vi "TCC.vi"() -> (2 "State out":string="Data: Load Thermal Calibration")   [LabVIEW 2024]
uses:
  DataCluster_TCAL.ctl
  <vilib>/vision/Image Controls.llb/IMAQ Image.ctl
  TCE_Config.ctl
  DataCluster.ctl
  <vilib>/userDefined/High Color/IMAQdx.ctl
  <vilib>/Utility/xml.llb/Write to XML File(string).vi
panel:
  out "OverlayTemp":bool=TRUE
  out "Pict Ring":i32(ring)
  in  "Save":bool
  out "Step":string="Step: 4\n\nCalculate temperature!"
  in  "Fixpoint Radius":i32=20 min=1 max=20
  in  "Cluster":T1={"Core"={"Current VI Reference"=refnum, "Close Panel on Exit?"=FALSE}, "Image Out"=refnum, "State"=0, "Points"={"Top Left"={"X"=0.0, "Y"=0.0}, "Top Right"={"X"=0.0, "Y"=0.0}, "Bottom Left"={"X"=0.0, "Y"=0.0}, "Bottom Right"={"X"=0.0, "Y"=0.0}, "x space 2"=0.0, "y space 2"=0.0, "x_space"=0.0, "y_space"=0.0, "Pixels"=[], "Fixpoint"={"X"=0.0, "Y"=0.0}}, "img_array"=[], "Temps"=[], "Temps_Array"=[], "Scan Area"=0.0, "Fixpoint Area"=0.0, "Config"={"Freezing"={"Cutoff"=2.0, "EndIndex"=2}}, "PCR Size"=0, "ImageCount"=0, "ShowGradient"=FALSE} {"Points"."Bottom Right"."Y" format="%.2f"; "Points"."Bottom Right"."X" format="%.2f"; "Points"."Top Left"."Y" format="%.2f"; "Points"."Top Left"."X" format="%.2f"; "Points"."Top Right"."Y" format="%.2f"; "Points"."Top Right"."X" format="%.2f"; "Points"."Bottom Left"."Y" format="%.2f"; "Points"."Bottom Left"."X" format="%.2f"; "Points"."Fixpoint"."Y" format="%.2f"; "Points"."Fixpoint"."X" format="%.2f"}
  in  "Display Mapping":u32(ring)=10 items=["Default"=10, "Most Significant Bits"=11, "Full Dynamic"=12, "Downshift"=13, "Given Range"=14, "90% Dynamic"=15, "Given Percent Range"=16]
  in  "Image":u32(slide) scale=0.0..242.0
  in  "Help":bool
  out "Tutorial":string="Step: 4\n\nCalculate temperature!"
  in  "Show All Points":bool
  in  "Well Radius":u32=50 min=1 max=100
  in  "PCR Size":u16(ring) items=["384 (24x16)", "96 (12x8)"]
  out "Points":T3[](array[typedef])=[{"X"=103.0, "Y"=94.0}, {"X"=158.04349, "Y"=93.521736}, {"X"=213.08696, "Y"=93.04348}, {"X"=268.13043, "Y"=92.565216}, {"X"=323.17392, "Y"=92.08696}, {"X"=378.2174, "Y"=91.608696}, {"X"=433.26086, "Y"=91.13043}, {"X"=488.30435, "Y"=90.652176}, {"X"=543.34784, "Y"=90.17391}, {"X"=598.39136, "Y"=89.69565}, {"X"=653.4348, "Y"=89.21739}, {"X"=708.4783, "Y"=88.73913}, {"X"=763.5217, "Y"=88.26087}, {"X"=818.56525, "Y"=87.78261}, {"X"=873.6087, "Y"=87.30435}, {"X"=928.6522, "Y"=86.82609}, {"X"=983.6957, "Y"=86.347824}, {"X"=1038.7391, "Y"=85.86957}, {"X"=1093.7827, "Y"=85.391304}, {"X"=1148.8262, "Y"=84.91304}, {"X"=1203.8696, "Y"=84.434784}, {"X"=1258.9131, "Y"=83.95652}, {"X"=1313.9565, "Y"=83.478264}, {"X"=1369.0, "Y"=83.0}, {"X"=103.46667, "Y"=149.06667}, {"X"=158.51015, "Y"=148.58841}, {"X"=213.55362, "Y"=148.11014}, {"X"=268.5971, "Y"=147.63188}, {"X"=323.6406, "Y"=147.15363}, {"X"=378.68408, "Y"=146.67535}, {"X"=433.72754, "Y"=146.1971}, {"X"=488.77103, "Y"=145.71884}, {"X"=543.8145, "Y"=145.24057}, {"X"=598.858, "Y"=144.76231}, {"X"=653.9015, "Y"=144.28406}, {"X"=708.94495, "Y"=143.8058}, {"X"=763.9884, "Y"=143.32753}, {"X"=819.0319, "Y"=142.84927}, {"X"=874.0754, "Y"=142.37102}, {"X"=929.1189, "Y"=141.89276}, {"X"=984.16235, "Y"=141.41449}, {"X"=1039.2058, "Y"=140.93623}, {"X"=1094.2493, "Y"=140.45798}, {"X"=1149.2928, "Y"=139.9797}, {"X"=1204.3363, "Y"=139.50145}, {"X"=1259.3798, "Y"=139.0232}, {"X"=1314.4232, "Y"=138.54492}, {"X"=1369.4667, "Y"=138.06667}, {"X"=103.933334, "Y"=204.13333}, {"X"=158.9768, "Y"=203.65506}, {"X"=214.0203, "Y"=203.17682}, {"X"=269.06375, "Y"=202.69855}, {"X"=324.10724, "Y"=202.22029}, {"X"=379.15073, "Y"=201.74203}, {"X"=434.19418, "Y"=201.26376}, {"X"=489.23767, "Y"=200.7855}, {"X"=544.2812, "Y"=200.30725}, {"X"=599.32465, "Y"=199.82898}, {"X"=654.36816, "Y"=199.35072}, {"X"=709.4116, "Y"=198.87247}, {"X"=764.4551, "Y"=198.3942}, {"X"=819.4986, "Y"=197.91594}, {"X"=874.54205, "Y"=197.43768}, {"X"=929.5856, "Y"=196.95941}, {"X"=984.629, "Y"=196.48116}, {"X"=1039.6725, "Y"=196.0029}, {"X"=1094.716, "Y"=195.52463}, {"X"=1149.7595, "Y"=195.04637}, {"X"=1204.803, "Y"=194.56812}, {"X"=1259.8464, "Y"=194.08984}, {"X"=1314.8899, "Y"=193.6116}, {"X"=1369.9333, "Y"=193.13333}, {"X"=104.4, "Y"=259.2}, {"X"=159.44348, "Y"=258.72174}, {"X"=214.48695, "Y"=258.24347}, {"X"=269.53043, "Y"=257.7652}, {"X"=324.5739, "Y"=257.28696}, {"X"=379.6174, "Y"=256.8087}, {"X"=434.66086, "Y"=256.33044}, {"X"=489.70435, "Y"=255.85217}, {"X"=544.74786, "Y"=255.37392}, {"X"=599.7913, "Y"=254.89565}, {"X"=654.83484, "Y"=254.41739}, {"X"=709.8783, "Y"=253.93913}, {"X"=764.92175, "Y"=253.46086}, {"X"=819.9653, "Y"=252.9826}, {"X"=875.0087, "Y"=252.50435}, {"X"=930.05225, "Y"=252.02608}, {"X"=985.0957, "Y"=251.54782}, {"X"=1040.1392, "Y"=251.06956}, {"X"=1095.1826, "Y"=250.59131}, {"X"=1150.2262, "Y"=250.11304}, {"X"=1205.2697, "Y"=249.63478}, {"X"=1260.3131, "Y"=249.15652}, {"X"=1315.3566, "Y"=248.67825}, {"X"=1370.4, "Y"=248.2}, {"X"=104.86667, "Y"=314.26666}, {"X"=159.91014, "Y"=313.7884}, {"X"=214.95363, "Y"=313.31012}, {"X"=269.9971, "Y"=312.83188}, {"X"=325.0406, "Y"=312.35364}, {"X"=380.08408, "Y"=311.87537}, {"X"=435.12753, "Y"=311.3971}, {"X"=490.17102, "Y"=310.91882}, {"X"=545.2145, "Y"=310.44058}, {"X"=600.258, "Y"=309.9623}, {"X"=655.30145, "Y"=309.48407}, {"X"=710.3449, "Y"=309.0058}, {"X"=765.38837, "Y"=308.52753}, {"X"=820.4319, "Y"=308.04926}, {"X"=875.47534, "Y"=307.571}, {"X"=930.51886, "Y"=307.09274}, {"X"=985.5623, "Y"=306.6145}, {"X"=1040.6058, "Y"=306.13623}, {"X"=1095.6493, "Y"=305.65796}, {"X"=1150.6929, "Y"=305.1797}, {"X"=1205.7363, "Y"=304.70145}, {"X"=1260.7798, "Y"=304.2232}, {"X"=1315.8232, "Y"=303.74493}, {"X"=1370.8667, "Y"=303.26666}, {"X"=105.333336, "Y"=369.3333}, {"X"=160.37682, "Y"=368.85504}, {"X"=215.42029, "Y"=368.3768}, {"X"=270.46378, "Y"=367.89853}, {"X"=325.50726, "Y"=367.42026}, {"X"=380.55075, "Y"=366.94202}, {"X"=435.5942, "Y"=366.46375}, {"X"=490.6377, "Y"=365.98547}, {"X"=545.68115, "Y"=365.50723}, {"X"=600.7247, "Y"=365.02896}, {"X"=655.7681, "Y"=364.5507}, {"X"=710.8116, "Y"=364.07245}, {"X"=765.85504, "Y"=363.59418}, {"X"=820.89856, "Y"=363.11594}, {"X"=875.942, "Y"=362.63766}, {"X"=930.98553, "Y"=362.1594}, {"X"=986.029, "Y"=361.68115}, {"X"=1041.0725, "Y"=361.20288}, {"X"=1096.116, "Y"=360.7246}, {"X"=1151.1595, "Y"=360.24637}, {"X"=1206.203, "Y"=359.7681}, {"X"=1261.2465, "Y"=359.28983}, {"X"=1316.2899, "Y"=358.81158}, {"X"=1371.3334, "Y"=358.3333}, {"X"=105.8, "Y"=424.4}, {"X"=160.84348, "Y"=423.92172}, {"X"=215.88696, "Y"=423.44348}, {"X"=270.93042, "Y"=422.9652}, {"X"=325.9739, "Y"=422.48694}, {"X"=381.0174, "Y"=422.0087}, {"X"=436.06085, "Y"=421.53043}, {"X"=491.10434, "Y"=421.05215}, {"X"=546.1478, "Y"=420.5739}, {"X"=601.19135, "Y"=420.09564}, {"X"=656.2348, "Y"=419.61737}, {"X"=711.27826, "Y"=419.13913}, {"X"=766.3217, "Y"=418.66086}, {"X"=821.36523, "Y"=418.18262}, {"X"=876.4087, "Y"=417.70435}, {"X"=931.4522, "Y"=417.22607}, {"X"=986.49567, "Y"=416.74783}, {"X"=1041.5392, "Y"=416.26956}, {"X"=1096.5826, "Y"=415.7913}, {"X"=1151.6262, "Y"=415.31305}, {"X"=1206.6697, "Y"=414.83478}, {"X"=1261.7131, "Y"=414.3565}, {"X"=1316.7566, "Y"=413.87827}, {"X"=1371.8, "Y"=413.4}, {"X"=106.26667, "Y"=479.46667}, {"X"=161.31015, "Y"=478.9884}, {"X"=216.35362, "Y"=478.51016}, {"X"=271.3971, "Y"=478.0319}, {"X"=326.44058, "Y"=477.55362}, {"X"=381.48407, "Y"=477.07538}, {"X"=436.52753, "Y"=476.5971}, {"X"=491.571, "Y"=476.11884}, {"X"=546.6145, "Y"=475.6406}, {"X"=601.658, "Y"=475.16232}, {"X"=656.7015, "Y"=474.68405}, {"X"=711.74493, "Y"=474.2058}, {"X"=766.7884, "Y"=473.72754}, {"X"=821.8319, "Y"=473.2493}, {"X"=876.87537, "Y"=472.77103}, {"X"=931.9189, "Y"=472.29276}, {"X"=986.96234, "Y"=471.8145}, {"X"=1042.0059, "Y"=471.33624}, {"X"=1097.0493, "Y"=470.85797}, {"X"=1152.0929, "Y"=470.37973}, {"X"=1207.1364, "Y"=469.90146}, {"X"=1262.1798, "Y"=469.4232}, {"X"=1317.2233, "Y"=468.94495}, {"X"=1372.2667, "Y"=468.46667}, {"X"=106.73333, "Y"=534.5333}, {"X"=161.77681, "Y"=534.05505}, {"X"=216.8203, "Y"=533.5768}, {"X"=271.86377, "Y"=533.0985}, {"X"=326.90726, "Y"=532.62024}, {"X"=381.95074, "Y"=532.142}, {"X"=436.9942, "Y"=531.66376}, {"X"=492.0377, "Y"=531.1855}, {"X"=547.0812, "Y"=530.7073}, {"X"=602.12463, "Y"=530.229}, {"X"=657.16815, "Y"=529.75073}, {"X"=712.2116, "Y"=529.27246}, {"X"=767.25507, "Y"=528.7942}, {"X"=822.2986, "Y"=528.3159}, {"X"=877.34204, "Y"=527.83765}, {"X"=932.38556, "Y"=527.3594}, {"X"=987.429, "Y"=526.88116}, {"X"=1042.4724, "Y"=526.4029}, {"X"=1097.516, "Y"=525.9246}, {"X"=1152.5594, "Y"=525.4464}, {"X"=1207.6029, "Y"=524.96814}, {"X"=1262.6464, "Y"=524.48987}, {"X"=1317.6898, "Y"=524.0116}, {"X"=1372.7333, "Y"=523.5333}, {"X"=107.2, "Y"=589.6}, {"X"=162.24348, "Y"=589.1217}, {"X"=217.28696, "Y"=588.64343}, {"X"=272.33044, "Y"=588.16516}, {"X"=327.37393, "Y"=587.6869}, {"X"=382.41742, "Y"=587.2087}, {"X"=437.46088, "Y"=586.7304}, {"X"=492.50436, "Y"=586.25214}, {"X"=547.54785, "Y"=585.7739}, {"X"=602.5913, "Y"=585.29565}, {"X"=657.6348, "Y"=584.8174}, {"X"=712.6783, "Y"=584.3391}, {"X"=767.72174, "Y"=583.86084}, {"X"=822.76526, "Y"=583.38257}, {"X"=877.8087, "Y"=582.9043}, {"X"=932.85223, "Y"=582.426}, {"X"=987.8957, "Y"=581.9478}, {"X"=1042.9391, "Y"=581.46954}, {"X"=1097.9827, "Y"=580.9913}, {"X"=1153.0261, "Y"=580.51306}, {"X"=1208.0696, "Y"=580.0348}, {"X"=1263.113, "Y"=579.5565}, {"X"=1318.1565, "Y"=579.07825}, {"X"=1373.2, "Y"=578.6}, {"X"=107.666664, "Y"=644.6666}, {"X"=162.71014, "Y"=644.18835}, {"X"=217.75363, "Y"=643.7101}, {"X"=272.7971, "Y"=643.2319}, {"X"=327.84058, "Y"=642.7536}, {"X"=382.88406, "Y"=642.2753}, {"X"=437.92752, "Y"=641.79706}, {"X"=492.971, "Y"=641.3188}, {"X"=548.0145, "Y"=640.8405}, {"X"=603.058, "Y"=640.3623}, {"X"=658.1015, "Y"=639.88403}, {"X"=713.14496, "Y"=639.40576}, {"X"=768.1884, "Y"=638.9275}, {"X"=823.23193, "Y"=638.4492}, {"X"=878.2754, "Y"=637.97095}, {"X"=933.3189, "Y"=637.49274}, {"X"=988.36237, "Y"=637.01447}, {"X"=1043.4058, "Y"=636.5362}, {"X"=1098.4493, "Y"=636.0579}, {"X"=1153.4928, "Y"=635.57965}, {"X"=1208.5363, "Y"=635.1014}, {"X"=1263.5797, "Y"=634.62317}, {"X"=1318.6232, "Y"=634.1449}, {"X"=1373.6666, "Y"=633.6666}, {"X"=108.13333, "Y"=699.73334}, {"X"=163.17682, "Y"=699.25507}, {"X"=218.22029, "Y"=698.7768}, {"X"=273.26376, "Y"=698.2986}, {"X"=328.30725, "Y"=697.8203}, {"X"=383.35074, "Y"=697.34204}, {"X"=438.3942, "Y"=696.8638}, {"X"=493.43768, "Y"=696.3855}, {"X"=548.4812, "Y"=695.9072}, {"X"=603.52466, "Y"=695.429}, {"X"=658.5682, "Y"=694.95074}, {"X"=713.61163, "Y"=694.4725}, {"X"=768.6551, "Y"=693.9942}, {"X"=823.6986, "Y"=693.5159}, {"X"=878.74207, "Y"=693.03766}, {"X"=933.7856, "Y"=692.55945}, {"X"=988.82904, "Y"=692.0812}, {"X"=1043.8724, "Y"=691.6029}, {"X"=1098.916, "Y"=691.12463}, {"X"=1153.9595, "Y"=690.64636}, {"X"=1209.0029, "Y"=690.1681}, {"X"=1264.0464, "Y"=689.6899}, {"X"=1319.0898, "Y"=689.2116}, {"X"=1374.1333, "Y"=688.73334}, {"X"=108.6, "Y"=754.8}, {"X"=163.64348, "Y"=754.3217}, {"X"=218.68697, "Y"=753.84344}, {"X"=273.73044, "Y"=753.36523}, {"X"=328.77393, "Y"=752.88696}, {"X"=383.8174, "Y"=752.4087}, {"X"=438.86087, "Y"=751.9304}, {"X"=493.90436, "Y"=751.45215}, {"X"=548.9478, "Y"=750.9739}, {"X"=603.99133, "Y"=750.49567}, {"X"=659.0348, "Y"=750.0174}, {"X"=714.07825, "Y"=749.5391}, {"X"=769.1217, "Y"=749.06085}, {"X"=824.1652, "Y"=748.5826}, {"X"=879.2087, "Y"=748.1043}, {"X"=934.2522, "Y"=747.6261}, {"X"=989.29565, "Y"=747.1478}, {"X"=1044.3391, "Y"=746.66956}, {"X"=1099.3827, "Y"=746.1913}, {"X"=1154.4261, "Y"=745.713}, {"X"=1209.4696, "Y"=745.23474}, {"X"=1264.5131, "Y"=744.75653}, {"X"=1319.5565, "Y"=744.27826}, {"X"=1374.6, "Y"=743.8}, {"X"=109.066666, "Y"=809.86664}, {"X"=164.11015, "Y"=809.38837}, {"X"=219.15363, "Y"=808.9101}, {"X"=274.1971, "Y"=808.4319}, {"X"=329.2406, "Y"=807.9536}, {"X"=384.2841, "Y"=807.47534}, {"X"=439.32755, "Y"=806.9971}, {"X"=494.37103, "Y"=806.5188}, {"X"=549.4145, "Y"=806.0405}, {"X"=604.458, "Y"=805.5623}, {"X"=659.50146, "Y"=805.08405}, {"X"=714.5449, "Y"=804.6058}, {"X"=769.5884, "Y"=804.1275}, {"X"=824.6319, "Y"=803.64923}, {"X"=879.67535, "Y"=803.17096}, {"X"=934.7189, "Y"=802.69275}, {"X"=989.7623, "Y"=802.2145}, {"X"=1044.8058, "Y"=801.7362}, {"X"=1099.8494, "Y"=801.25793}, {"X"=1154.8928, "Y"=800.77966}, {"X"=1209.9363, "Y"=800.3014}, {"X"=1264.9797, "Y"=799.8232}, {"X"=1320.0232, "Y"=799.3449}, {"X"=1375.0667, "Y"=798.86664}, {"X"=109.53333, "Y"=864.93335}, {"X"=164.57681, "Y"=864.4551}, {"X"=219.6203, "Y"=863.9768}, {"X"=274.66376, "Y"=863.4986}, {"X"=329.70724, "Y"=863.0203}, {"X"=384.75073, "Y"=862.54205}, {"X"=439.7942, "Y"=862.0638}, {"X"=494.83768, "Y"=861.5855}, {"X"=549.88116, "Y"=861.10724}, {"X"=604.9247, "Y"=860.629}, {"X"=659.96814, "Y"=860.15076}, {"X"=715.0116, "Y"=859.6725}, {"X"=770.05505, "Y"=859.1942}, {"X"=825.0986, "Y"=858.71594}, {"X"=880.142, "Y"=858.2377}, {"X"=935.18555, "Y"=857.75946}, {"X"=990.229, "Y"=857.2812}, {"X"=1045.2725, "Y"=856.8029}, {"X"=1100.316, "Y"=856.32465}, {"X"=1155.3595, "Y"=855.8464}, {"X"=1210.403, "Y"=855.3681}, {"X"=1265.4464, "Y"=854.8899}, {"X"=1320.4899, "Y"=854.4116}, {"X"=1375.5333, "Y"=853.93335}, {"X"=110.0, "Y"=920.0}, {"X"=165.04349, "Y"=919.5217}, {"X"=220.08696, "Y"=919.04346}, {"X"=275.13043, "Y"=918.56525}, {"X"=330.17392, "Y"=918.087}, {"X"=385.2174, "Y"=917.6087}, {"X"=440.26086, "Y"=917.13043}, {"X"=495.30435, "Y"=916.65216}, {"X"=550.34784, "Y"=916.1739}, {"X"=605.39136, "Y"=915.6957}, {"X"=660.4348, "Y"=915.2174}, {"X"=715.4783, "Y"=914.73914}, {"X"=770.5217, "Y"=914.26086}, {"X"=825.56525, "Y"=913.7826}, {"X"=880.6087, "Y"=913.3043}, {"X"=935.6522, "Y"=912.8261}, {"X"=990.6957, "Y"=912.34784}, {"X"=1045.7391, "Y"=911.86957}, {"X"=1100.7827, "Y"=911.3913}, {"X"=1155.8262, "Y"=910.913}, {"X"=1210.8696, "Y"=910.43475}, {"X"=1265.9131, "Y"=909.95654}, {"X"=1320.9565, "Y"=909.4783}, {"X"=1376.0, "Y"=909.0}] {"Y" format="%.2f"; "X" format="%.2f"}
  out "State":i32=3
  in  "Previous":bool
  in  "Next":bool
  in  "Path":path caption="Image Path"
  out "Image":T2(plugin-control)
  # "hints \nPress F1 or F2 to cycle through the steps\nUse the Mouse Wheel to zoom in and out"
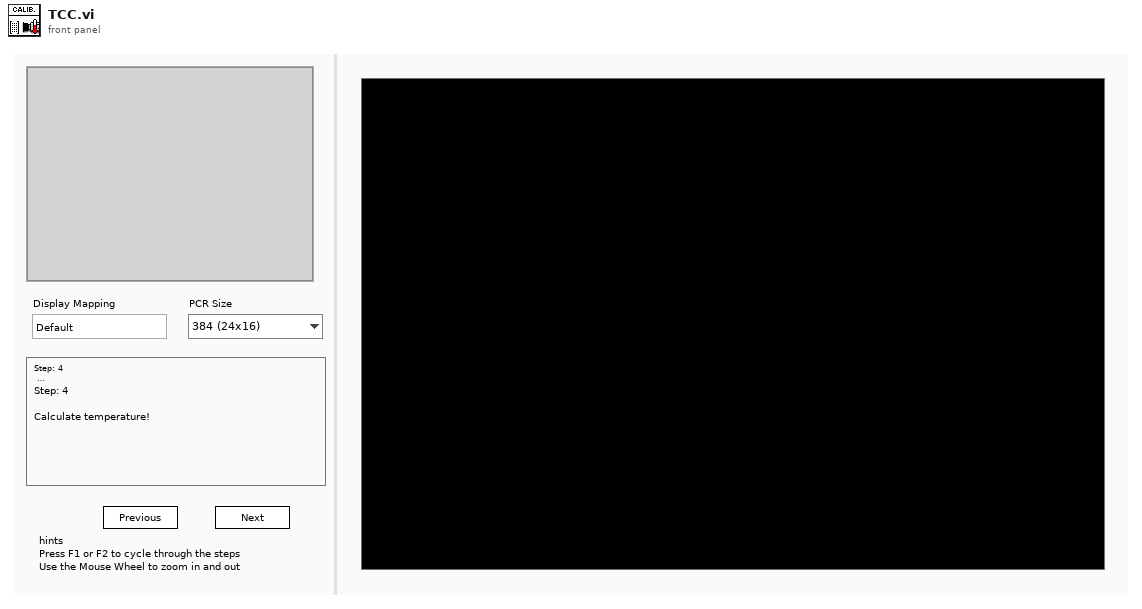
[diagram p1: front panel]
types:
  T1 = typedef "DataCluster_TCAL.ctl" = cluster{"Core":cluster{"Current VI Reference":refnum<vi>, "Close Panel on Exit?":bool}, "Image Out":T2, "State":i32, "Points":cluster{"Top Left":T3, "Top Right":T3, "Bottom Left":T3, "Bottom Right":T3, "x space 2":dbl, "y space 2":sgl, "x_space":sgl, "y_space":sgl, "Pixels":cluster{"X":i32, "Y":i32}[][], "Fixpoint":T3}, "img_array":T2[], "Temps":dbl[], "Temps_Array":dbl[][], "Scan Area":dbl, "Fixpoint Area":dbl, "Config":T4, "PCR Size":u16, "ImageCount":i32, "ShowGradient":bool}
  T2 = typedef "IMAQ Image.ctl" = refnum<image>
  T3 = typedef "IMAQ Point" = cluster{"X":sgl, "Y":sgl}
  T4 = typedef "TCE_Config.ctl" = cluster{"Freezing":cluster{"Cutoff":dbl, "EndIndex":i32}}
  T5 = enum32{"Invalid", "Standard", "Closed", "Hidden", "Minimized", "Maximized"}
  T6 = enum32{"invalid app kind", "Development System", "Run Time System", "Student Edition", "Embedded LabVIEW", "Evaluation", "Custom"}
  T7 = cluster{"Global Rectangle":i32[], "Contours":cluster{"Contour Type":u32, "ROI Type":u32, "Points":i32[]}[]}
  T8 = typedef "DataCluster.ctl" = cluster{"Core":cluster{"Current VI Reference":refnum<vi>, "Close Panel on Exit?":bool, "Exit":bool, "Initialized?":bool}, "Connections":cluster{"cDAQ":cluster{"Task":refnum<k21>, "Connected":bool, "Active":bool, "ID":string}, "Camera":cluster{"Session":T9, "Connected":bool, "Active":bool, "Placeholder":T2}, "PSU":cluster{"Port":refnum<visa-resource-name>, "Connected":bool, "Active":bool}, "Arduino":cluster{"Port":refnum<visa-resource-name>, "Connected":bool, "Active":bool}}, "Data Acquisition":cluster{"Setup":cluster{"Label":string, "Operator":string, "Notes":string, "TempGrad":dbl, "TargetTemp":dbl, "Sample Volume":dbl}, "Camera":cluster{"Image":T2, "Save Image":T2, "Image Frequency":i32, "Rectangle":T10, "Calibration":cluster{"Top Left":T3, "Top Right":T3, "Bottom Left":T3, "Bottom Right":T3, "Fixpoint":T3, "Scan Area":dbl, "Fixpoint Area":dbl, "Well Pixels":cluster{"X":i32, "Y":i32}[][], "Valid":bool}, "FocusPos":u32, "Display Mapping":u32, "Camera Mode":u32}, "Thermistor":cluster{"Sample Size":i32, "Calibration":cluster{"B0.100":dbl[], "R25":dbl[], "c":dbl[][], "State":bool[], "V_S":dbl, "R_S":dbl}, "Timing Mode":i32}, "Partition":cluster{"Data":string[][], "Cell Label":string, "Cell Color":u32, "Height":i32, "Width":i32, "Grid":string[][]}, "Queue":cluster{"Size":i32, "Queue":refnum<queue>}, "Sample Rate":i32, "Active":bool, "Ready":bool, "Graph Mode":u16, "Gradient Buffer":i32}, "Control":cluster{"Sample Rate":i32, "PID gains":cluster{"proportional gain (Kc)":dbl, "integral time (Ti, min)":dbl, "derivative time (Td, min)":dbl}}, "Manual Temp Control":cluster{"TargetTemp":dbl, "Mode":u16, "Active":bool}}
  T9 = typedef "IMAQdx.ctl" = refnum<k21>
  T10 = typedef "IMAQ Rectangle" = cluster{"Left":i32, "Top":i32, "Right":i32, "Bottom":i32, "Rotation":dbl}
  T11 = enum16{"open", "replace", "create", "open or create", "replace or create", "replace or create with confirmation"}
  T12 = typedef "ROI Descriptor" = cluster{"Global Rectangle":i32[], "Contours":cluster{"ID":enum32{"External", "Internal"}, "Type":u32, "Coordinates":i32[]}[]}
  T13 = typedef "Image Type" = u32
  T14 = cluster{"Current VI Reference":refnum<vi>, "Close Panel on Exit?":bool}
  T15 = cluster{"Top Left":T3, "Top Right":T3, "Bottom Left":T3, "Bottom Right":T3, "x space 2":dbl, "y space 2":sgl, "x_space":sgl, "y_space":sgl, "Pixels":cluster{"X":i32, "Y":i32}[][], "Fixpoint":T3}
  T16 = cluster{"Top Left":T3, "Top Right":T3, "Bottom Left":T3, "Bottom Right":T3, "Fixpoint":T3, "Scan Area":dbl, "Fixpoint Area":dbl, "Well Pixels":cluster{"X":i32, "Y":i32}[][], "Valid":bool}
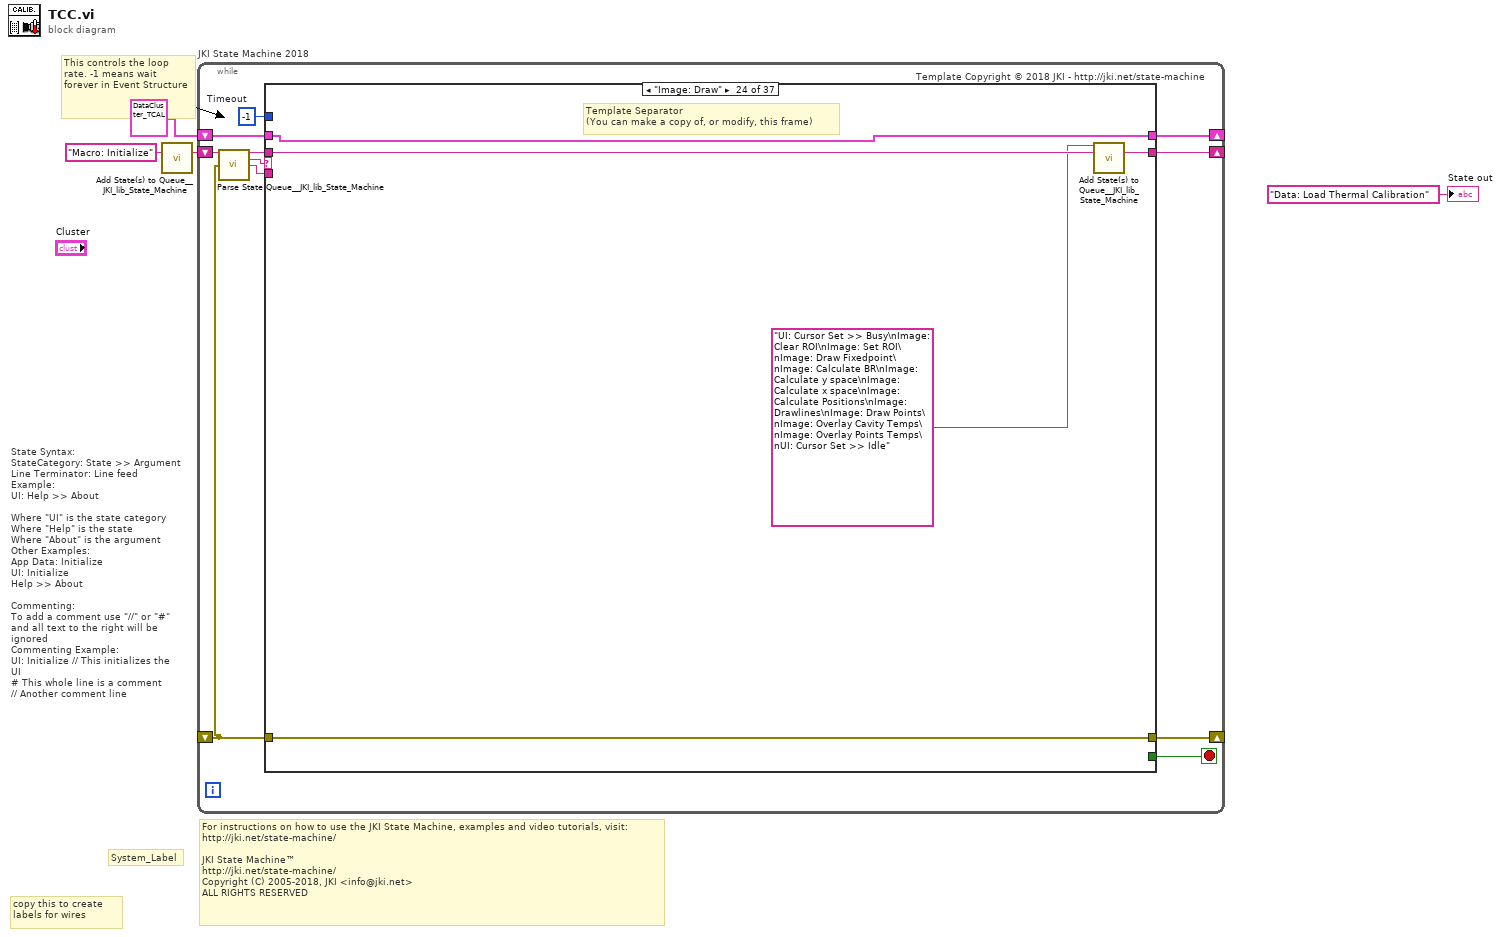
[diagram p0: block diagram]
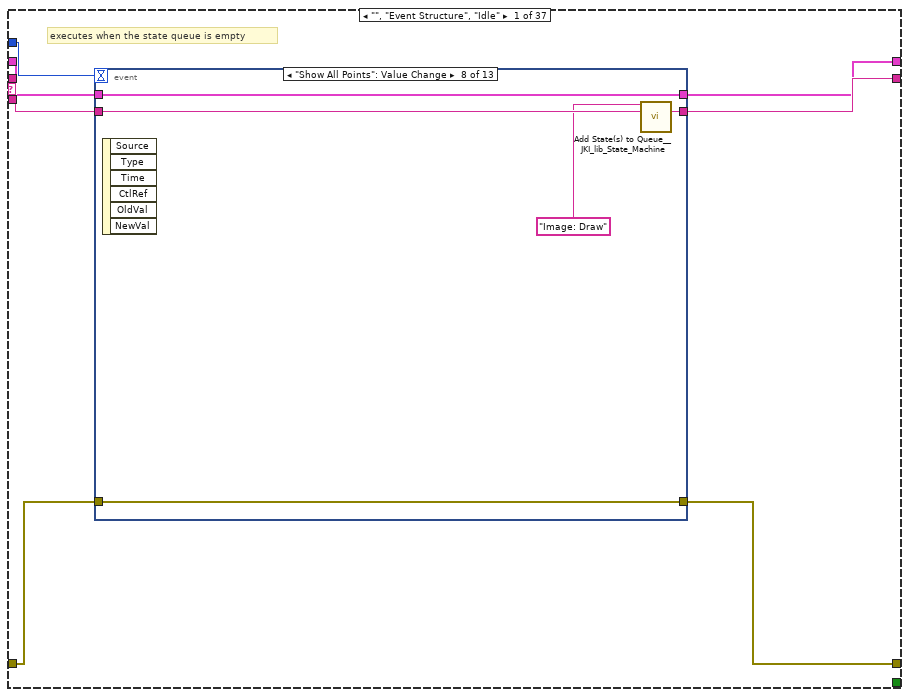
[diagram p2: hidden frame]
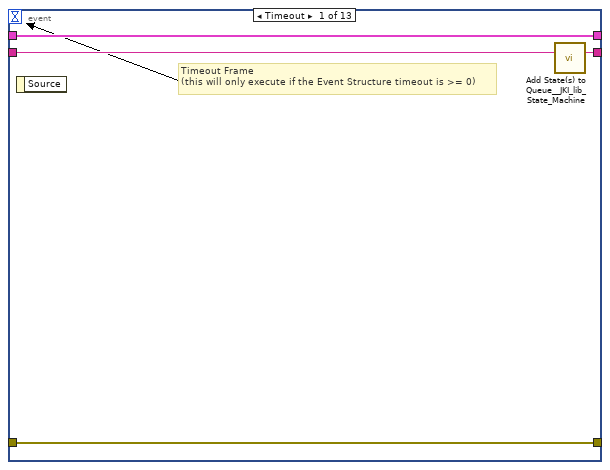
[diagram p3: hidden frame]
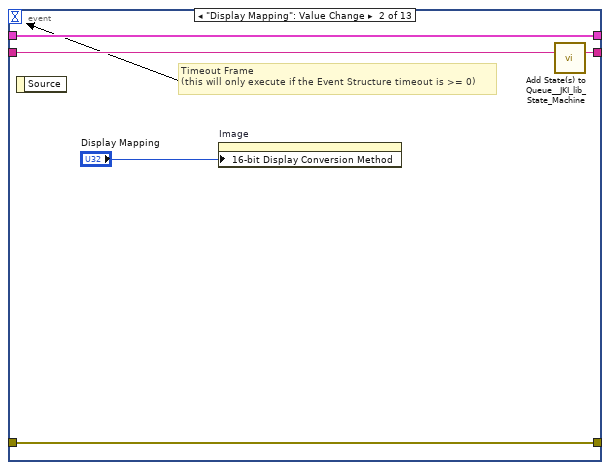
[diagram p4: hidden frame]
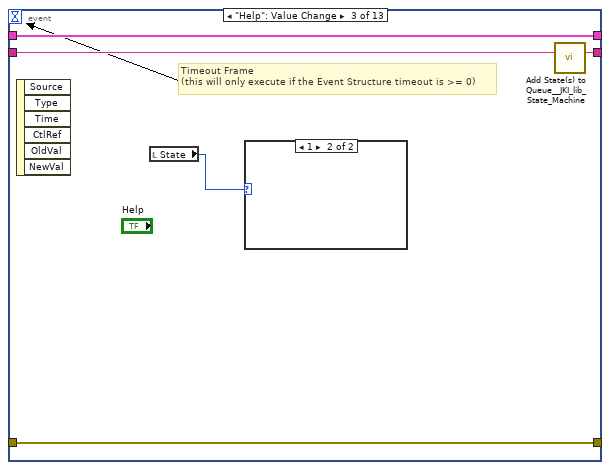
[diagram p5: hidden frame]
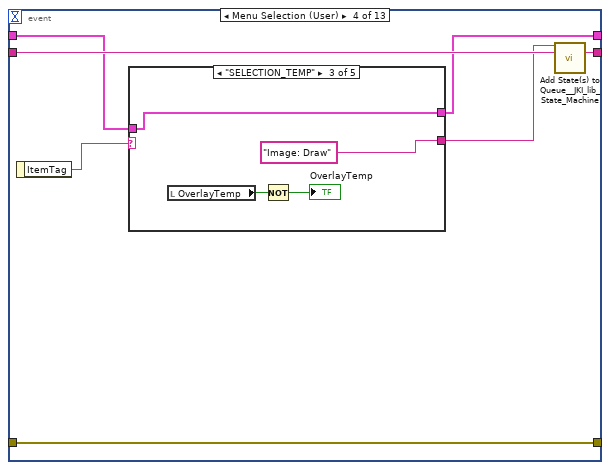
[diagram p7: hidden frame]
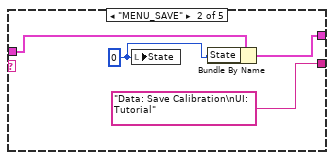
[diagram p9: hidden frame]
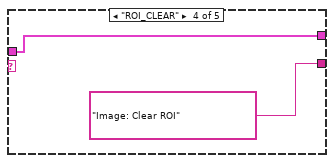
[diagram p10: hidden frame]
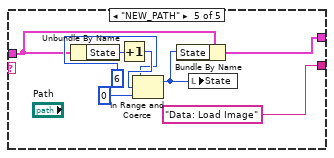
[diagram p11: hidden frame]
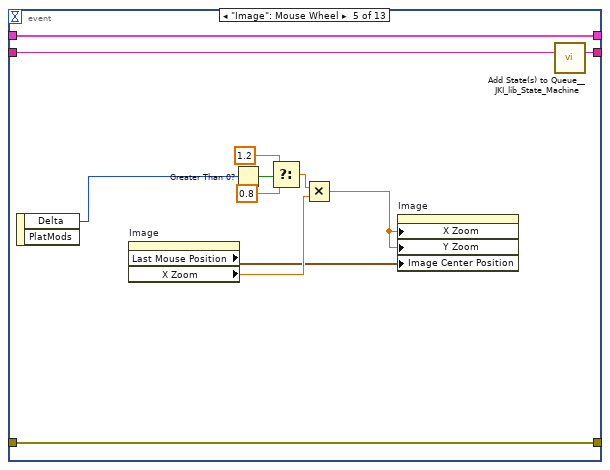
[diagram p12: hidden frame]
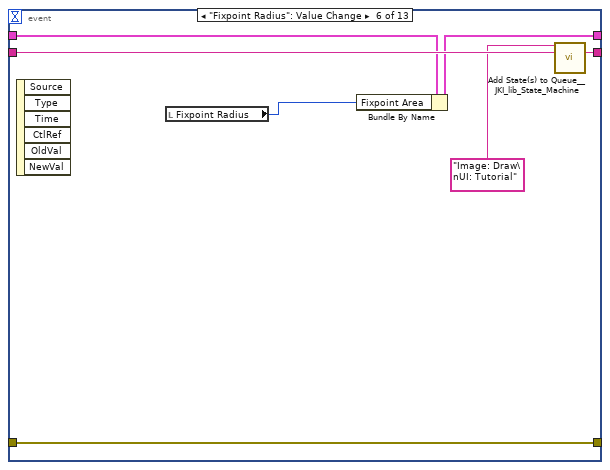
[diagram p13: hidden frame]
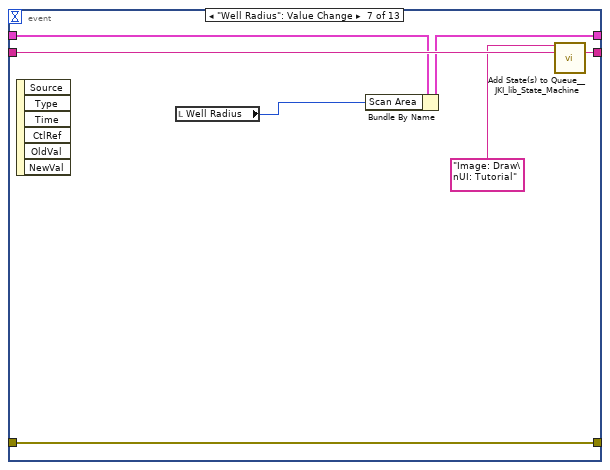
[diagram p14: hidden frame]
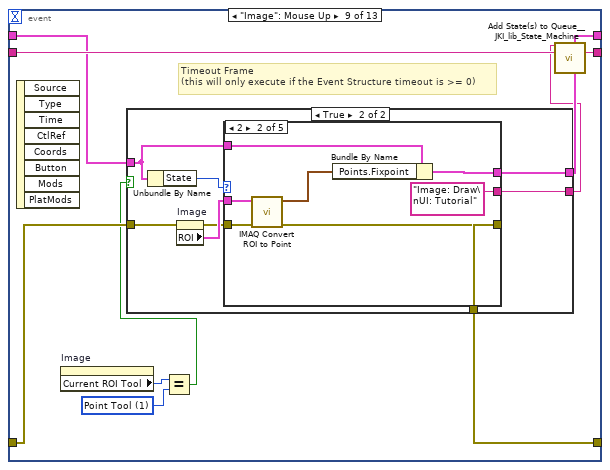
[diagram p15: hidden frame]
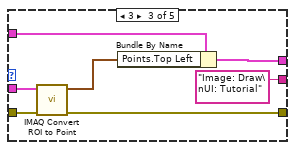
[diagram p18: hidden frame]
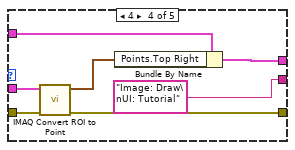
[diagram p19: hidden frame]
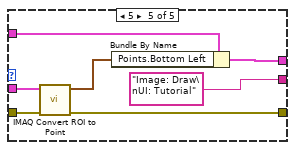
[diagram p20: hidden frame]
diagram:
  # "For instructions on how to use the JKI State Machine, examples and video tutorials, visit:\nhttp://jki.net/state-machine/\n\nJKI State Machine™\nhttp://jki.net/state-machine/\nCopyright (C) 2005-2018, JKI <info@jki.net>\nALL RIGHTS RESERVED"
  # "State Syntax:\nStateCategory: State >> Argument\nLine Terminator: Line feed\nExample:\nUI: Help >> About\n\nWhere \"UI\" is the state category\nWhere \"Help\" is the state\nWhere \"About\" is the argument\nOther Examples:\nApp Data: Initialize\nUI: Initialize\nHelp >> About\n\nCommenting:\nTo add a comment use \"//\" or \"#\" and all text to the right will be ignored\nCommenting Example:\nUI: Initialize // This initializes the UI\n# This whole line is a comment\n// Another comment line"
  # "copy this to create labels for wires"
  # "This controls the loop rate. -1 means wait forever in Event Structure"
  # "System_Label"
  n1 = call <vilib>:"Add State(s) to Queue__JKI_lib_State_Machine.vi"("State(s) in (\"\")"="Macro: Initialize") -> ("States Out"=w4:string)  [unwired: 14 in]
  n2 = while "JKI State Machine 2018" {
    shift-right: [w8] -> _
    shift-left: T1 {"Core"={"Current VI Reference"=refnum, "Close Panel on Exit?"=FALSE}, "Image Out"=refnum, "State"=0, "Points"={"Top Left"={"X"=0.0, "Y"=0.0}, "Top Right"={"X"=0.0, "Y"=0.0}, "Bottom Left"={"X"=0.0, "Y"=0.0}, "Bottom Right"={"X"=0.0, "Y"=0.0}, "x space 2"=0.0, "y space 2"=0.0, "x_space"=0.0, "y_space"=0.0, "Pixels"=[], "Fixpoint"={"X"=0.0, "Y"=0.0}}, "img_array"=[], "Temps"=[], "Temps_Array"=[], "Scan Area"=0.0, "Fixpoint Area"=0.0, "Config"={"Freezing"={"Cutoff"=2.0, "EndIndex"=2}}, "PCR Size"=0, "ImageCount"=0, "ShowGradient"=FALSE} ("output cluster") -> [w7]
    shift-right: [w11] -> _
    shift-left: _ -> [w5]
    shift-right: [w10] -> _
    shift-left: w4 -> [w12]
    stop <- w9 stop-if-true
    w6 = -1  # Timeout
    # "Template Copyright © 2018 JKI - http://jki.net/state-machine"
    n3 = call <vilib>:"Parse State Queue__JKI_lib_State_Machine.vi"("State Queue"=w12, "Error In (no error)"=w5) -> ("Remaining States"=w14:string, "Current State"=w15:string, "Arguments"=w13:string)  [unwired: 11 in]
    n4 = case shown="\"Image: Draw\"" w15 {
      selector: w15 -> [_ _ w185 _ _ _ _ _ _ _ _ _ _ _ _ _ _ _ _ _ _ _ _ _ _ _ _ _ _ _ _ _ _ _ _ _ _]
      tunnel: w14 -> [w22 w184 w189 w208 w214 w219 w223 w236 w267 w272 w290 w303 w344 w372 w393 w414 w432 w498 w509 w578 w583 w594 w598 w603 w608 w628 w645 w650 w664 w682 w702 w720 w731 w759 w824 w838 w869]
      tunnel: w13 -> [_ _ _ _ _ _ _ _ _ _ _ _ _ _ _ _ _ w493 w503 _ _ _ _ _ _ _ _ _ _ _ _ _ _ w757 _ _ _]
      tunnel: w7 -> [w20 w181 w187 w201 w211 w217 w220 w226 w264 w268 _ w299 w341 w370 w390 w412 w419 w496 w505 w575 w580 w591 w595 w600 w605 w609 w643 w648 w662 w673 w693 w711 w729 w755 w811 w834 w858]
      tunnel: [w19 w182 w191 w205 errorcluster {"status"=FALSE, "code"=0, "source"=""} ("error out") w216 w221 w230 w261 w270 w281 w300 w338 w353 w391 w411 w430 w494 w506 w576 w581 w592 w596 w601 w606 w626 w638 w647 w659 w680 w700 w718 w724 w752 w821 w836 w867] -> w11
      tunnel: w5 -> [w18 w182 w190 w205 w210 w216 w221 w233 w261 w270 w282 w301 w337 w369 w391 w411 w430 w495 w507 w576 w581 w592 w596 w601 w606 w626 w638 w647 w660 w680 w700 w718 w728 w753 w821 w836 w867]
      tunnel: [w21 w183 w188 w207 w213 w218 w222 w235 w266 w271 w289 w302 w343 w371 w392 w413 w431 w497 w508 w577 w582 w593 w597 w602 w607 w627 w644 w649 w663 w681 w701 w719 w730 w758 w823 w837 w868] -> w10
      tunnel: [_ _ _ _ _ TRUE _ _ _ _ _ _ _ _ _ _ _ _ _ _ _ _ _ _ _ _ _ _ _ _ _ _ _ _ _ _ _] -> w9
      tunnel: [w17 w181 w187 w206 w211 w217 w220 w234 w265 w268 w288 w295 w341 w370 w390 w412 w419 w496 w505 w575 w580 w591 w595 w600 w605 w609 w643 w648 w662 w672 w692 w710 w729 w755 w810 w834 w858] -> w8
      tunnel: w6 -> [w16 _ _ _ _ _ _ _ _ _ _ _ _ _ _ _ _ _ _ _ _ _ _ _ _ _ _ _ _ _ _ _ _ _ _ _ _]
      frame "", "Event Structure", "Idle" {
        # "executes when the state queue is empty"
        n5 = event shown="[7] \"Show All Points\": Value Change" {
          selector: _ -> [_ _ _ _ _ _ _ _ _ _ _ _ _]
          dyn-events: _ -> [_ _ _ _ _ _ _ _ _ _ _ _ _]
          timeout: w16 -> [_ _ _ _ _ _ _ _ _ _ _ _ _]
          tunnel: w22 -> [w26 w31 w36 w43 w74 w81 w88 w93 w103 w155 w167 w173 w180]
          tunnel: [w25 w30 w35 w42 w73 w80 w87 w92 w102 w154 w166 w172 w179] -> w21
          tunnel: w20 -> [w23 w28 w33 w38 w71 w78 w85 w90 w100 w153 w165 w170 w176]
          tunnel: [w24 w29 w34 w41 w72 w79 w86 w91 w98 w150 w162 w171 w178] -> w19
          tunnel: w18 -> [w24 w29 w34 w41 w72 w79 w86 w91 w101 w150 w162 w171 w178]
          tunnel: [w23 w28 w33 w39 w71 w76 w83 w90 w99 w151 w163 w170 w174] -> w17
          event Timeout {
            # "Timeout Frame\n(this will only execute if the Event Structure timeout is >= 0)"
            n6 = event-data() -> ()  [unwired: 1 in, 1 out]
            n7 = call <vilib>:"Add State(s) to Queue__JKI_lib_State_Machine.vi"("State(s) in (\"\")"=w26) -> ("States Out"=w25:string)  [unwired: 14 in]
          }
          event "Display Mapping": Value Change {
            # "Timeout Frame\n(this will only execute if the Event Structure timeout is >= 0)"
            n8 = event-data() -> ()  [unwired: 1 in, 1 out]
            n9 = property on="Image" class="ImageControl"("16-bit Display Conversion Method"="Display Mapping") -> ()  [unwired: 2 in, 2 out]
            n10 = call <vilib>:"Add State(s) to Queue__JKI_lib_State_Machine.vi"("State(s) in (\"\")"=w31) -> ("States Out"=w30:string)  [unwired: 14 in]
          }
          event "Help": Value Change {
            # "Timeout Frame\n(this will only execute if the Event Structure timeout is >= 0)"
            n11 = event-data() -> ()  [unwired: 1 in, 6 out]
            n12 = local read "State"() -> (w32:i32)
            n13 = case shown="1" w32 {
              frame 0, Default {
              }
              frame 1 {
              }
            }
            n14 = call <vilib>:"Add State(s) to Queue__JKI_lib_State_Machine.vi"("State(s) in (\"\")"=w36) -> ("States Out"=w35:string)  [unwired: 14 in]
          }
          event Menu Selection (User) {
            n15 = event-data() -> ("ItemTag"=w37:string)  [unwired: 1 in]
            n16 = case shown="\"SELECTION_TEMP\"" w37 {
              tunnel: [_ "Data: Save Calibration\nUI: Tutorial" "Image: Draw" "Image: Clear ROI" "Data: Load Image" ("State(s) in Front (\"\")")] -> w40
              tunnel: [w44 w47 w52 w54 w57] -> w39
              tunnel: w38 -> [w44 w48 w52 w54 w56]
              frame "False", Default {
              }
              frame "MENU_SAVE" {
                w45 = 0 ("lower limit")
                n17 = local write "State"(w45) -> ()
                n18 = Bundle By Name(cluster=w48, "State"=w45) -> (w47:T1)
              }
              frame "SELECTION_TEMP" {
                n19 = local read "OverlayTemp"() -> (w49:bool)
                n20 = Not(x=w49) -> (.not. x?=→"OverlayTemp":bool)
              }
              frame "ROI_CLEAR" {
              }
              frame "NEW_PATH" {
                n21 = Unbundle By Name(w56) -> ("State"=w61:i32)
                n22 = Increment(x=w61) -> (x+1=w60:i32)
                n23 = In Range and Coerce(upper limit=6, x=w60, lower limit=0) -> (coerced(x)=w55:i32)  [unwired: 1 out]
                n24 = Bundle By Name(cluster=w56, "State"=w55) -> (w57:T1)
                n25 = local write "State"(w55) -> ()
              }
            }
            n26 = call <vilib>:"Add State(s) to Queue__JKI_lib_State_Machine.vi"("State(s) in Front (\"\")"=w40, "State(s) in (\"\")"=w43) -> ("States Out"=w42:string)  [unwired: 13 in]
          }
          event "Image": Mouse Wheel {
            n27 = event-data() -> ("Delta"=w70:i32)  [unwired: 1 in, 1 out]
            n28 = property on="Image" class="ImageControl"() -> ("Last Mouse Position"=w64:cluster{"X":i32, "Y":i32}, "X Zoom"=w65:sgl)  [unwired: 2 in, 2 out]
            n29 = Greater Than 0?(x=w70) -> (x > 0?=w69:bool)
            n30 = Select(t=1.2, s=w69, f=0.8) -> (s? t:f=w66:dbl)
            n31 = Multiply(x=w66, y=w65) -> (x*y=w63:dbl)
            n32 = property on="Image" class="ImageControl"("X Zoom"=w63, "Y Zoom"=w63, "Image Center Position"=w64) -> ()  [unwired: 2 in, 2 out]
            n33 = call <vilib>:"Add State(s) to Queue__JKI_lib_State_Machine.vi"("State(s) in (\"\")"=w74) -> ("States Out"=w73:string)  [unwired: 14 in]
          }
          event "Fixpoint Radius": Value Change {
            n34 = event-data() -> ()  [unwired: 1 in, 6 out]
            n35 = local read "Fixpoint Radius"() -> (w75:i32)
            n36 = Bundle By Name(cluster=w78, "Fixpoint Area"=w75) -> (w76:T1)
            n37 = call <vilib>:"Add State(s) to Queue__JKI_lib_State_Machine.vi"("State(s) in Front (\"\")"="Image: Draw\nUI: Tutorial" ("State(s) in Front (\"\")"), "State(s) in (\"\")"=w81) -> ("States Out"=w80:string)  [unwired: 13 in]
          }
          event "Well Radius": Value Change {
            n38 = event-data() -> ()  [unwired: 1 in, 6 out]
            n39 = local read "Well Radius"() -> (w82:u32)
            n40 = Bundle By Name(cluster=w85, "Scan Area"=w82) -> (w83:T1)
            n41 = call <vilib>:"Add State(s) to Queue__JKI_lib_State_Machine.vi"("State(s) in Front (\"\")"="Image: Draw\nUI: Tutorial" ("State(s) in Front (\"\")"), "State(s) in (\"\")"=w88) -> ("States Out"=w87:string)  [unwired: 13 in]
          }
          event "Show All Points": Value Change {
            n42 = event-data() -> ()  [unwired: 1 in, 6 out]
            n43 = call <vilib>:"Add State(s) to Queue__JKI_lib_State_Machine.vi"("State(s) in Front (\"\")"="Image: Draw" ("State(s) in Front (\"\")"), "State(s) in (\"\")"=w93) -> ("States Out"=w92:string)  [unwired: 13 in]
          }
          event "Image": Mouse Up {
            w96 = u32 1 items=["Zoom Tool"=8, "Selection Tool"=0, "Pan Tool"=9, "Point Tool"=1, "Line Tool"=2, "Rectangle Tool"=3, "Rotated Rectangle Tool"=12, "Polyline Tool"=10, "Polygon Tool"=5, "Freehand Tool"=11, "Closed Freehand Tool"=6, "Ellipse Tool"=4, "Annulus Tool"=7] ("Current ROI Tool")
            # "Timeout Frame\n(this will only execute if the Event Structure timeout is >= 0)"
            n44 = event-data() -> ()  [unwired: 1 in, 8 out]
            n45 = property on="Image" class="ImageControl"() -> ("Current ROI Tool"=w97:u32)  [unwired: 2 in, 2 out]
            n46 = Equal?(x=w97, y=w96) -> (x = y?=w95:bool)
            n47 = case shown="True" w95 {
              tunnel: w101 -> [w105 w110]
              tunnel: w100 -> [w104 w109]
              tunnel: [w104 w108] -> w99
              tunnel: [w105 w107] -> w98
              tunnel: [_ w106] -> w94
              frame False {
              }
              frame True {
                n48 = Unbundle By Name(w109) -> ("State"=w113:i32)
                n49 = property on="Image" class="ImageControl"(error in=w110) -> (error out=w111:errorcluster, "ROI"=w112:T7)  [unwired: 1 in, 1 out]
                n50 = case shown="2" w113 {
                  tunnel: w112 -> [_ w121 w128 w136 w143]
                  tunnel: w111 -> [w114 w120 w127 w135 w142]
                  tunnel: w109 -> [w115 w117 w124 w134 w141]
                  tunnel: [w115 w118 w125 w133 w140] -> w108
                  tunnel: [w114 w119 w126 w131 w138] -> w107
                  tunnel: [_ "Image: Draw\nUI: Tutorial" "Image: Draw\nUI: Tutorial" "Image: Draw\nUI: Tutorial" "Image: Draw\nUI: Tutorial"] -> w106
                  frame -1, Default {
                  }
                  frame 2 {
                    n51 = call "IMAQ Convert ROI to Point"("error in (no error)"=w120, "ROI Descriptor"=w121) -> ("error out"=w119:errorcluster, "Point"=w122:T3)  [unwired: 7 in]
                    n52 = Bundle By Name(cluster=w117, "Points.Fixpoint"=w122) -> (w118:T1)
                  }
                  frame 3 {
                    n53 = call "IMAQ Convert ROI to Point"("error in (no error)"=w127, "ROI Descriptor"=w128) -> ("error out"=w126:errorcluster, "Point"=w129:T3)  [unwired: 7 in]
                    n54 = Bundle By Name(cluster=w124, "Points.Top Left"=w129) -> (w125:T1)
                  }
                  frame 4 {
                    n55 = call "IMAQ Convert ROI to Point"("error in (no error)"=w135, "ROI Descriptor"=w136) -> ("error out"=w131:errorcluster, "Point"=w132:T3)  [unwired: 7 in]
                    n56 = Bundle By Name(cluster=w134, "Points.Top Right"=w132) -> (w133:T1)
                  }
                  frame 5 {
                    n57 = call "IMAQ Convert ROI to Point"("error in (no error)"=w142, "ROI Descriptor"=w143) -> ("error out"=w138:errorcluster, "Point"=w139:T3)  [unwired: 7 in]
                    n58 = Bundle By Name(cluster=w141, "Points.Bottom Left"=w139) -> (w140:T1)
                  }
                }
              }
            }
            n59 = call <vilib>:"Add State(s) to Queue__JKI_lib_State_Machine.vi"("State(s) in Front (\"\")"=w94, "State(s) in (\"\")"=w103) -> ("States Out"=w102:string)  [unwired: 13 in]
          }
          event "Next": Value Change {
            # "Timeout Frame\n(this will only execute if the Event Structure timeout is >= 0)"
            n60 = event-data() -> ()  [unwired: 1 in, 6 out]
            n61 = Unbundle By Name(w153) -> ("State"=w152:i32)
            n62 = Increment(x=w152) -> (x+1=w148:i32)
            n63 = In Range and Coerce(upper limit=6, x=w148, lower limit=0) -> (coerced(x)=w145:i32)  [unwired: 1 out]
            n64 = property on="Image" class="ImageControl"("Zoom to Fit Mode"=TRUE) -> ()  [unwired: 2 in, 2 out]
            n65 = local write "State"(w145) -> ()
            n66 = Bundle By Name(cluster=w153, "State"=w145) -> (w151:T1)
            n67 = call <vilib>:"Add State(s) to Queue__JKI_lib_State_Machine.vi"("State(s) in Front (\"\")"="UI: Tutorial\nImage: Set ROI" ("f"), "State(s) in (\"\")"=w155) -> ("States Out"=w154:string)  [unwired: 13 in]
          }
          event "Previous": Value Change {
            # "Timeout Frame\n(this will only execute if the Event Structure timeout is >= 0)"
            n68 = event-data() -> ()  [unwired: 1 in, 6 out]
            n69 = Unbundle By Name(w165) -> ("State"=w164:i32)
            n70 = Decrement(x=w164) -> (x-1=w159:i32)
            n71 = In Range and Coerce(upper limit=6, x=w159, lower limit=0) -> (coerced(x)=w160:i32)  [unwired: 1 out]
            "State" <- w160
            n72 = Bundle By Name(cluster=w165, "State"=w160) -> (w163:T1)
            n73 = property on="Image" class="ImageControl"("Zoom to Fit Mode"=TRUE) -> ()  [unwired: 2 in, 2 out]
            n74 = call <vilib>:"Add State(s) to Queue__JKI_lib_State_Machine.vi"("State(s) in Front (\"\")"="UI: Tutorial\nImage: Set ROI" ("f"), "State(s) in (\"\")"=w167) -> ("States Out"=w166:string)  [unwired: 13 in]
          }
          event Panel Close? {
            (unwired) TRUE ("Discard?")
            # "Close Panel button (pressed) Event\n(this executes Macro: Exit to terminate the VI)"
            n75 = event-data() -> ()  [unwired: 1 in, 1 out]
            n76 = event-data("Discard?"=TRUE) -> ()  [unwired: 1 in, 1 out]
            n77 = call <vilib>:"Add State(s) to Queue__JKI_lib_State_Machine.vi"("State(s) in Front (\"\")"="Macro: Exit", "State(s) in (\"\")"=w173) -> ("States Out"=w172:string)  [unwired: 13 in]
          }
          event "Save": Value Change {
            w175 = 0 ("lower limit")
            # "Close Panel button (pressed) Event\n(this executes Macro: Exit to terminate the VI)"
            n78 = event-data() -> ()  [unwired: 1 in, 6 out]
            n79 = local write "State"(w175) -> ()
            n80 = Bundle By Name(cluster=w176, "State"=w175) -> (w174:T1)
            n81 = call <vilib>:"Add State(s) to Queue__JKI_lib_State_Machine.vi"("State(s) in Front (\"\")"="Data: Save Calibration\nUI: Tutorial", "State(s) in (\"\")"=w180) -> ("States Out"=w179:string)  [unwired: 13 in]
          }
        }
      }
      frame "---------- Core ----------" {
        # "Do not put any code in this frame.\n(it is a separator no-op)"
        n82 = call <vilib>:"Add State(s) to Queue__JKI_lib_State_Machine.vi"("State(s) in (\"\")"=w184) -> ("States Out"=w183:string)  [unwired: 14 in]
      }
      frame Default {
        w194 = 42 items=["No error", "Argument error", "Memory is full", "Out of zone", "End of file", "File already open", "Generic file I/O error", "File not found", "File permission error", "Disk is full", "Duplicate path", "Too many files open", "System feature not enabled", "Resource file not found", "Cannot add resource", "Resource not found", "Image not found", "Image memory error", "Pen does not exist", "Config type invalid", "Config token not found", "Config parse error", "Config memory error", "Bad external code format", "Bad external code offset", "External code not present", "Null window", "Destroy window error", "Null menu", "Print aborted", "Bad print record", "Print driver error", "Windows error during printing", "Memory error during printing", "Print dialog error", "Generic print error", "Invalid device refnum", "Device not found", "Device parameter error", "Device unit error", "Cannot open device", "Device call aborted", "Generic error", "Cancelled by user", "Object ID too low", "Object ID too high", "Object not in heap", "Unknown heap", "Unknown object (invalid DefProc)", "Unknown object (DefProc not in table)", "Message out of range", "Invalid (null) method", "Unknown message", "Manager call not supported", "Bad address", "Network operation in progress", "Network operation timed out", "Connection is busy", "Network attribute not supported", "Network error", "Address in use", "System out of memory", "Connection aborted", "Connection refused", "Not connected", "Already connected", "Connection closed", "Initialization error (interapplication manager)", "Bad occurrence", "Wait on unbound occurrence handler", "Occurrence queue overflow", "Datalog type conflict", "Unused", "Unrecognized type (interapplication manager)", "Memory corrupt", "Failed to make temporary DLL", "Old CIN version", "Drag socket not found", "Failed to load drop-object", "Failed to register OLE object", "Failed to release OLE object", "Format specifier type mismatch", "Unknown format specifier", "Too few format specifiers", "Too many format specifiers", "Scan failed", "Newer CIN version", "Error converting to variant", "Runtime menu error", "Password tampered", "Variant attribute not found", "Incompatible variant data type", "Event data is not available", "Event Store is not present", "Occurrence is not found", "Event Queue is not created", "Event info is not available", "Refnum passed is NULL", "Error retrieving Class GUID", "Error retrieving CoClass GUID", "Error retrieving TypeLib GUID.", "Bad built application magic bytes.", "Specific driver is different from the specific driver associated with the Logical Name.", "There is no session opened to the class driver.", "Max Error", "MAX - Error with config objects", "MAX - Error loading configuration", "MAX - Group not supported"]
        # "Current State"
        # "Do not delete, rename, or modify this frame.\n(this is used to capture unhandled states and typos)"
        # "Handle mistyped state name (developer tool)"
        n83 = Format Into String(format string="Software Exception: Unhandled State \"%s\"." ("message"), error in=w190, w185) -> (resulting string=w193:string, error out=w192:errorcluster)  [unwired: 1 in]
        n84 = call <vilib>:"Error Cluster From Error Code.vi"("show call chain? (False)"=TRUE, "error in (no error)"=w192, "error message (\"\")"=w193, "error code (0)"=w194) -> ("error out"=w191:errorcluster)  [unwired: 5 in]
        n85 = call <vilib>:"Add State(s) to Queue__JKI_lib_State_Machine.vi"("State(s) in (\"\")"=w189) -> ("States Out"=w188:string)  [unwired: 14 in]
      }
      frame "Initialize Core Data" {
        # "Do not delete, rename, or modify this frame.\n(this is used to determine panel behavior on exit)"
        # "originally closed?"
        # "exe?"
        # "If panel starts closed or is an EXE, then close it when we exit"
        n86 = property class="App"() -> ("App.Kind"=w204:T6)  [unwired: 2 in, 2 out]
        n87 = control-ref of="Current VI Reference"() -> (w199:refnum<vi>)
        n88 = property class="VI"() -> ("FP.State"=w198:T5)  [unwired: 2 in, 2 out]
        n89 = Equal?(x=w198, y=T5."Closed" ("Front Panel Window:State")) -> (x = y?=w196:bool)
        n90 = Equal?(x=w204, y=T6."Run Time System" ("Application:Kind")) -> (x = y?=w202:bool)
        n91 = Or(x=w196, y=w202) -> (x .or. y?=w200:bool)
        n92 = Bundle By Name(cluster=w201, "Core.Current VI Reference"=w199, "Core.Close Panel on Exit?"=w200) -> (w206:T1)
        n93 = call <vilib>:"Add State(s) to Queue__JKI_lib_State_Machine.vi"("State(s) in (\"\")"=w208) -> ("States Out"=w207:string)  [unwired: 14 in]
      }
      frame "Error Handler" {
        # "Unhandled Error -- Display it"
        # "Handle any errors here.\nYou can also output any states to clean-up after errors occur"
        # "Clear error"
        n94 = call <vilib>:"General Error Handler.vi"("error in (no error)"=w210) -> ()  [unwired: 10 in, 5 out]
        n95 = call <vilib>:"Add State(s) to Queue__JKI_lib_State_Machine.vi"("State(s) in Front (\"\")"="/* Post Error States", "State(s) in (\"\")"=w214) -> ("States Out"=w213:string)  [unwired: 13 in]
      }
      frame "Exit" {
        # "Do not put any code in this frame.\n(No errors that occur here will be handled.)"
        n96 = call <vilib>:"Add State(s) to Queue__JKI_lib_State_Machine.vi"("State(s) in (\"\")"=w219) -> ("States Out"=w218:string)  [unwired: 14 in]
      }
      frame "---------- Data ----------" {
        # "Do not put any code in this frame.\n(It is a separator no-op. You can make a copy of this frame to create a new Data frame)"
        n97 = call <vilib>:"Add State(s) to Queue__JKI_lib_State_Machine.vi"("State(s) in (\"\")"=w223) -> ("States Out"=w222:string)  [unwired: 14 in]
      }
      frame "Data: Load Image" {
        # "Do not put any code in this frame.\n(It is a separator no-op. You can make a copy of this frame to create a new Data frame)"
        n98 = call "CalibrationImageLoadPrompt.vi"() -> ("cancel?"=w228:bool, "selected path"=w224:path)  [unwired: 10 in]
        n99 = Empty String/Path?(string/path=w224) -> (empty?=w232:bool)
        n100 = Or(x=w232, y=w228) -> (x .or. y?=w229:bool)
        n101 = local write "Path"(w224) -> ()
        n102 = case shown="False" w229 {
          tunnel: w233 -> [w244 w259]
          tunnel: [w253 w259] -> w230
          tunnel: w224 -> [w252 _]
          tunnel: [w246 _] -> w231
          tunnel: ["Data: Load Calibration\nImage: Draw\nUI: Tutorial" ("State(s) in Front (\"\")") "" ("State(s) in Front (\"\")")] -> w227
          tunnel: w226 -> [w238 w257]
          tunnel: [w237 w256] -> w225
          frame False {
            w248 = T13 7 items=["Grayscale (U8)", "Grayscale (I16)", "Grayscale (SGL)", "Complex (CSG)", "RGB (U32)", "HSL (U32)", "RGB (U64)", "Grayscale (U16)"] ("Image Type")
            n103 = Unbundle By Name(w238) -> ("State"=w242:i32)
            n104 = Increment(x=w242) -> (x+1=w241:i32)
            n105 = call "IMAQ Create"("Image Name"="img_in", "Image Type"=w248, "error in (no error)"=w244) -> ("New Image"=w250:T2, "error out"=w251:errorcluster)  [unwired: 2 in]
            n106 = In Range and Coerce(upper limit=6, x=w241, lower limit=0) -> (coerced(x)=w237:i32)  [unwired: 1 out]
            n107 = call "IMAQ ReadFile 2"("File Path"=w252, "error in (no error)"=w251, "Image"=w250) -> ("error out"=w249:errorcluster, "Image Out"=w247:T2)  [unwired: 4 in, 3 out]
            n108 = local write "State"(w237) -> ()
            n109 = call "IMAQ Clear Overlay"("error in (no error)"=w249, "Image"=w247) -> ("error out"=w255:errorcluster, "Image Out"=w246:T2)  [unwired: 8 in]
            "Image" <- w246
            n110 = property on="Image" class="ImageControl"(error in=w255, "ROI"=T7 {"Global Rectangle"=[], "Contours"=[]}) -> (error out=w253:errorcluster)  [unwired: 1 in, 1 out]
          }
          frame True {
            n111 = Unbundle By Name(w257) -> ("State"=w256:i32)
          }
        }
        n112 = Bundle By Name(cluster=w226, "Image Out"=w231, "State"=w225) -> (w234:T1)
        n113 = call <vilib>:"Add State(s) to Queue__JKI_lib_State_Machine.vi"("State(s) in Front (\"\")"=w227, "State(s) in (\"\")"=w236) -> ("States Out"=w235:string)  [unwired: 13 in]
      }
      frame "Data: Set Image" {
        # "Do not put any code in this frame.\n(It is a separator no-op. You can make a copy of this frame to create a new Data frame)"
        n114 = Unbundle By Name(w264) -> ("img_array"=w263:T2[])
        n115 = Index Array(array=w263, index="Image") -> (element=w260:T2)
        n116 = Bundle By Name(cluster=w264, "Image Out"=w260) -> (w265:T1)
        n117 = call <vilib>:"Add State(s) to Queue__JKI_lib_State_Machine.vi"("State(s) in (\"\")"=w267) -> ("States Out"=w266:string)  [unwired: 14 in]
      }
      frame "Data: Show Img" {
        # "Do not put any code in this frame.\n(It is a separator no-op. You can make a copy of this frame to create a new Data frame)"
        n118 = Unbundle By Name(w268) -> ("Image Out"=w269:T2)
        n119 = local write "Image"(w269) -> ()
        n120 = call <vilib>:"Add State(s) to Queue__JKI_lib_State_Machine.vi"("State(s) in (\"\")"=w272) -> ("States Out"=w271:string)  [unwired: 14 in]
      }
      frame "Data: Initialize" {
        w283 = dbl[][] []  # Temps_Array
        w284 = dbl[] []  # Temps
        w285 = T2[] []  # img_array
        w279 = 0  # State
        w287 = T14 {"Current VI Reference"=refnum, "Close Panel on Exit?"=FALSE}  # Core
        # "Initialize the shift-register data, here.\n(data names are defined by what you wire into the bundle function)"
        n121 = call <vilib>:"Application Directory.vi"() -> ("Application Directory"=w275:path)
        n122 = Build Path(base path=w275, name or relative path=path "TCam.ini") -> (appended path=w273:path)
        n123 = call "TCam_Calibration_LoadSettings.vi"("error in (no error)"=w282, "path"=w273) -> ("error out"=w281:errorcluster, "Fixpoint Area"=w277:dbl, "Scan Area"=w278:dbl, "Points"=w280:T15)  [unwired: 6 in]
        n124 = local write "Fixpoint Radius"(w277) -> ()
        n125 = local write "Well Radius"(w278) -> ()
        n126 = local write "State"(w279) -> ()
        n127 = Bundle(cluster=T1 {"Core"={"Current VI Reference"=refnum, "Close Panel on Exit?"=FALSE}, "Image Out"=refnum, "State"=0, "Points"={"Top Left"={"X"=0.0, "Y"=0.0}, "Top Right"={"X"=0.0, "Y"=0.0}, "Bottom Left"={"X"=0.0, "Y"=0.0}, "Bottom Right"={"X"=0.0, "Y"=0.0}, "x space 2"=0.0, "y space 2"=0.0, "x_space"=0.0, "y_space"=0.0, "Pixels"=[], "Fixpoint"={"X"=0.0, "Y"=0.0}}, "img_array"=[], "Temps"=[], "Temps_Array"=[], "Scan Area"=0.0, "Fixpoint Area"=0.0, "Config"={"Freezing"={"Cutoff"=2.0, "EndIndex"=2}}, "PCR Size"=0, "ImageCount"=0, "ShowGradient"=FALSE} ("output cluster"), "Core"=w287, "Image Out"=T2 refnum, "State"=w279, "Points"=w280, "img_array"=w285, "Temps"=w284, "Temps_Array"=w283) -> (w288:T1)  [unwired: 6 in]
        n128 = call <vilib>:"Add State(s) to Queue__JKI_lib_State_Machine.vi"("State(s) in (\"\")"=w290) -> ("States Out"=w289:string)  [unwired: 14 in]
      }
      frame "Data: Load Calibration" {
        # "Initialize the shift-register data, here.\n(data names are defined by what you wire into the bundle function)"
        n129 = local read "Path"() -> (w298:path)
        n130 = Strip Path(path=w298) -> (stripped path=w292:path)  [unwired: 1 out]
        n131 = Strip Path(path=w292) -> (stripped path=w291:path)  [unwired: 1 out]
        n132 = Build Path(base path=w291, name or relative path=path "TCC.cal") -> (appended path=w296:path)
        n133 = call <vilib>:"Check if File or Folder Exists.vi"("path"=w296) -> ("file or folder exists?"=w294:bool, "dup path"=w293:path)  [unwired: 8 in, 1 out]
        n134 = case shown="True" w294 {
          tunnel: w301 -> [w304 w313]
          tunnel: [w304 w312] -> w300
          tunnel: w299 -> [w305 w309]
          tunnel: [w305 w307] -> w295
          tunnel: w293 -> [_ w306]
          frame False {
          }
          frame True {
            n135 = call "TCam_Calibration_LoadSettings.vi"("error in (no error)"=w313, "path"=w306) -> ("error out"=w312:errorcluster, "Fixpoint Area"=w310:dbl, "Scan Area"=w311:dbl, "Points"=w308:T15)  [unwired: 6 in]
            n136 = local write "Fixpoint Radius"(w310) -> ()
            n137 = local write "Well Radius"(w311) -> ()
            n138 = Bundle By Name(cluster=w309, "Points"=w308) -> (w307:T1)
          }
        }
        n139 = call <vilib>:"Add State(s) to Queue__JKI_lib_State_Machine.vi"("State(s) in (\"\")"=w303) -> ("States Out"=w302:string)  [unwired: 14 in]
      }
      frame "Data: Cleanup" {
        # "Cleanup any data and references, here.\n(this is called automatically, by the Macro: Exit)"
        n140 = Unbundle By Name(w341) -> ("Points.Top Left"=w334:T3, "Points.Top Right"=w333:T3, "Points.Bottom Left"=w332:T3, "Points.Bottom Right"=w331:T3, "Points.Fixpoint"=w327:T3, "Core.Current VI Reference"=w342:refnum<vi>)
        n141 = local read "Fixpoint Radius"() -> (w325:i32)
        n142 = local read "Well Radius"() -> (w330:u32)
        n143 = Unbundle By Name(T8 {"Core"={"Current VI Reference"=refnum, "Close Panel on Exit?"=FALSE, "Exit"=FALSE, "Initialized?"=FALSE}, "Connections"={"cDAQ"={"Task"="", "Connected"=FALSE, "Active"=FALSE, "ID"=""}, "Camera"={"Session"="", "Connected"=FALSE, "Active"=FALSE, "Placeholder"=refnum}, "PSU"={"Port"="", "Connected"=FALSE, "Active"=FALSE}, "Arduino"={"Port"="", "Connected"=FALSE, "Active"=FALSE}}, "Data Acquisition"={"Setup"={"Label"="", "Operator"="", "Notes"="", "TempGrad"=1.0, "TargetTemp"=1.0, "Sample Volume"=1.0}, "Camera"={"Image"=refnum, "Save Image"=refnum, "Image Frequency"=20, "Rectangle"={"Left"=0, "Top"=0, "Right"=0, "Bottom"=0, "Rotation"=0.0}, "Calibration"={"Top Left"={"X"=0.0, "Y"=0.0}, "Top Right"={"X"=0.0, "Y"=0.0}, "Bottom Left"={"X"=0.0, "Y"=0.0}, "Bottom Right"={"X"=0.0, "Y"=0.0}, "Fixpoint"={"X"=0.0, "Y"=0.0}, "Scan Area"=5.0, "Fixpoint Area"=0.0, "Well Pixels"=[], "Valid"=FALSE}, "FocusPos"=0, "Display Mapping"=10, "Camera Mode"=10}, "Thermistor"={"Sample Size"=1, "Calibration"={"B0.100"=[], "R25"=[], "c"=[], "State"=[], "V_S"=5.0, "R_S"=100.0}, "Timing Mode"=14713}, "Partition"={"Data"=[], "Cell Label"="", "Cell Color"=0, "Height"=10, "Width"=16, "Grid"=[]}, "Queue"={"Size"=1, "Queue"=refnum}, "Sample Rate"=20, "Active"=FALSE, "Ready"=FALSE, "Graph Mode"=0, "Gradient Buffer"=2}, "Control"={"Sample Rate"=1, "PID gains"={"proportional gain (Kc)"=1.0, "integral time (Ti, min)"=0.01, "derivative time (Td, min)"=0.0}}, "Manual Temp Control"={"TargetTemp"=1.0, "Mode"=0, "Active"=FALSE}} ("Default values")) -> ("Data Acquisition.Camera.Calibration"=w323:T16)
        n144 = Bundle(cluster=w323, "Top Left"=w334, "Top Right"=w333, "Bottom Left"=w332, "Bottom Right"=w331, "Fixpoint"=w327, "Scan Area"=w330, "Fixpoint Area"=w325, "Well Pixels"=cluster{"X":i32, "Y":i32}[][] [], "Valid"=FALSE) -> (w335:T16)
        n145 = call <vilib>:"Application Directory.vi"() -> ("Application Directory"=w322:path)
        n146 = Build Path(base path=w322, name or relative path=path "TCam.ini") -> (appended path=w320:path)
        n147 = call <vilib>:"Check if File or Folder Exists.vi"("error in (no error)"=w337, "path"=w320) -> ("error out"=w317:errorcluster, "file or folder exists?"=w319:bool, "dup path"=w318:path)  [unwired: 7 in]
        n148 = case shown="False" w319 {
          tunnel: w318 -> [w345 w349]
          tunnel: w317 -> [w347 w350]
          tunnel: [w346 w350] -> w316
          tunnel: [w345 w349] -> w315
          frame False {
            n149 = Open/Create/Replace File(file path (use dialog)=w345, error in=w347, operation (0:open)=T11."create") -> (error out=w346:errorcluster)  [unwired: 3 in, 2 out]
          }
          frame True {
          }
        }
        n150 = Flatten To XML(6:w335) -> (2:w314:string)
        n151 = call-poly <vilib>:"Write to XML File.vi"("error in (no error)"=w316, "XML Input"=w314, "XML File Path"=w315) -> ("error out"=w336:errorcluster)  [unwired: 6 in, 2 out]
        n152 = local read "Image"() -> (w326:T2)
        n153 = Close Reference(reference=w342, error in (no error)=w336) -> (error out=w339:errorcluster)
        n154 = call "IMAQ Dispose"("All Images? (No)"=FALSE, "Image"=w326, "error in (no error)"=w339) -> ("error out"=w338:errorcluster)  [unwired: 3 in]
        n155 = call <vilib>:"Add State(s) to Queue__JKI_lib_State_Machine.vi"("State(s) in (\"\")"=w344) -> ("States Out"=w343:string)  [unwired: 14 in]
      }
      frame "Data: Save Calibration" {
        # "Cleanup any data and references, here.\n(this is called automatically, by the Macro: Exit)"
        n156 = local read "Fixpoint Radius"() -> (w359:i32)
        n157 = Unbundle By Name(w370) -> ("Points.Top Left"=w367:T3, "Points.Top Right"=w366:T3, "Points.Bottom Left"=w365:T3, "Points.Bottom Right"=w364:T3, "Points.Fixpoint"=w360:T3)
        n158 = local read "Well Radius"() -> (w363:u32)
        n159 = Unbundle By Name(T8 {"Core"={"Current VI Reference"=refnum, "Close Panel on Exit?"=FALSE, "Exit"=FALSE, "Initialized?"=FALSE}, "Connections"={"cDAQ"={"Task"="", "Connected"=FALSE, "Active"=FALSE, "ID"=""}, "Camera"={"Session"="", "Connected"=FALSE, "Active"=FALSE, "Placeholder"=refnum}, "PSU"={"Port"="", "Connected"=FALSE, "Active"=FALSE}, "Arduino"={"Port"="", "Connected"=FALSE, "Active"=FALSE}}, "Data Acquisition"={"Setup"={"Label"="", "Operator"="", "Notes"="", "TempGrad"=1.0, "TargetTemp"=1.0, "Sample Volume"=1.0}, "Camera"={"Image"=refnum, "Save Image"=refnum, "Image Frequency"=20, "Rectangle"={"Left"=0, "Top"=0, "Right"=0, "Bottom"=0, "Rotation"=0.0}, "Calibration"={"Top Left"={"X"=0.0, "Y"=0.0}, "Top Right"={"X"=0.0, "Y"=0.0}, "Bottom Left"={"X"=0.0, "Y"=0.0}, "Bottom Right"={"X"=0.0, "Y"=0.0}, "Fixpoint"={"X"=0.0, "Y"=0.0}, "Scan Area"=5.0, "Fixpoint Area"=0.0, "Well Pixels"=[], "Valid"=FALSE}, "FocusPos"=0, "Display Mapping"=10, "Camera Mode"=10}, "Thermistor"={"Sample Size"=1, "Calibration"={"B0.100"=[], "R25"=[], "c"=[], "State"=[], "V_S"=5.0, "R_S"=100.0}, "Timing Mode"=14713}, "Partition"={"Data"=[], "Cell Label"="", "Cell Color"=0, "Height"=10, "Width"=16, "Grid"=[]}, "Queue"={"Size"=1, "Queue"=refnum}, "Sample Rate"=20, "Active"=FALSE, "Ready"=FALSE, "Graph Mode"=0, "Gradient Buffer"=2}, "Control"={"Sample Rate"=1, "PID gains"={"proportional gain (Kc)"=1.0, "integral time (Ti, min)"=0.01, "derivative time (Td, min)"=0.0}}, "Manual Temp Control"={"TargetTemp"=1.0, "Mode"=0, "Active"=FALSE}} ("Default values")) -> ("Data Acquisition.Camera.Calibration"=w357:T16)
        n160 = Bundle(cluster=w357, "Top Left"=w367, "Top Right"=w366, "Bottom Left"=w365, "Bottom Right"=w364, "Fixpoint"=w360, "Scan Area"=w363, "Fixpoint Area"=w359, "Well Pixels"=cluster{"X":i32, "Y":i32}[][] [], "Valid"=FALSE) -> (w368:T16)
        n161 = local read "Path"() -> (w356:path)
        n162 = Strip Path(path=w356) -> (stripped path=w352:path)  [unwired: 1 out]
        n163 = Strip Path(path=w352) -> (stripped path=w351:path)  [unwired: 1 out]
        n164 = call "CalibrationSavePrompt.vi"("Root Path"=w351) -> ("selected path"=w355:path, "cancel?"=w354:bool)
        n165 = case shown="False" w354 {
          tunnel: w369 -> [w376 w389]
          tunnel: [w375 w389] -> w353
          tunnel: w368 -> [w374 _]
          tunnel: w355 -> [w373 _]
          frame False {
            n166 = call <vilib>:"Check if File or Folder Exists.vi"("error in (no error)"=w376, "path"=w373) -> ("error out"=w380:errorcluster, "file or folder exists?"=w382:bool, "dup path"=w381:path)  [unwired: 7 in]
            n167 = case shown="False" w382 {
              tunnel: w381 -> [w383 w387]
              tunnel: w380 -> [w385 w388]
              tunnel: [w384 w388] -> w379
              tunnel: [w383 w387] -> w378
              frame False {
                n168 = Open/Create/Replace File(file path (use dialog)=w383, error in=w385, operation (0:open)=T11."create") -> (error out=w384:errorcluster)  [unwired: 3 in, 2 out]
              }
              frame True {
              }
            }
            n169 = Flatten To XML(6:w374) -> (2:w377:string)
            n170 = call-poly <vilib>:"Write to XML File.vi"("error in (no error)"=w379, "XML Input"=w377, "XML File Path"=w378) -> ("error out"=w375:errorcluster)  [unwired: 6 in, 2 out]
          }
          frame True {
          }
        }
        n171 = call <vilib>:"Add State(s) to Queue__JKI_lib_State_Machine.vi"("State(s) in (\"\")"=w372) -> ("States Out"=w371:string)  [unwired: 14 in]
      }
      frame "---------- UI ----------" {
        # "Do not put any code in this frame.\n(It is a separator no-op. You can make a copy of this frame to create a new UI frame)"
        n172 = call <vilib>:"Add State(s) to Queue__JKI_lib_State_Machine.vi"("State(s) in (\"\")"=w393) -> ("States Out"=w392:string)  [unwired: 14 in]
      }
      frame "UI: Initialize" {
        w395 = u32 0 items=["Grayscale", "Binary", "Gradient", "Rainbow", "Temperature", "User Defined", "Binary 16 Bit", "Gradient 16 Bit", "Rainbow 16 Bit", "Temperature 16 Bit", "User Defined 16 Bit"] ("Palette:Palette Type")
        w400 = T13 4 items=["Grayscale (U8)", "Grayscale (I16)", "Grayscale (SGL)", "Complex (CSG)", "RGB (U32)", "HSL (U32)", "RGB (U64)", "Grayscale (U16)"] ("Image Type")
        w408 = u32 1 items=["Zoom Tool"=8, "Selection Tool"=0, "Pan Tool"=9, "Point Tool"=1, "Line Tool"=2, "Rectangle Tool"=3, "Rotated Rectangle Tool"=12, "Polyline Tool"=10, "Polygon Tool"=5, "Freehand Tool"=11, "Closed Freehand Tool"=6, "Ellipse Tool"=4, "Annulus Tool"=7] ("Current ROI Tool")
        w409 = u32 15 items=["Default"=10, "Most Significant Bits"=11, "Full Dynamic"=12, "Downshift"=13, "Given Range"=14, "90% Dynamic"=15, "Given Percent Range"=16] ("16-bit Display Mapping:Conversion Method")
        # "Initialize the User Interface, here.\n(this is called automatically, by the Macro: Init)"
        n173 = call <vilib>:"Application Directory.vi"() -> ("Application Directory"=w404:path)
        n174 = Path To String(path=w404) -> (string=w406:string)
        n175 = call "IMAQ Create"("Image Name"="placeholder_img_TCC", "Image Type"=w400) -> ("New Image"=w403:T2)  [unwired: 3 in, 1 out]
        n176 = Concatenate Strings(w406, "\\camera_placeholder.png") -> (w405:string)
        n177 = String To Path(string=w405) -> (path=w407:path)
        n178 = call "IMAQ ReadFile 2"("Use File Path Image Type"=FALSE, "File Path"=w407, "Image"=w403) -> ("Image Out"=w398:T2)  [unwired: 4 in, 4 out]
        n179 = local write "OverlayTemp"(FALSE ("OverlayTemp")) -> ()
        n180 = property on="Image" class="ImageControl"("Current ROI Tool"=w408, "Palette Type"=w395) -> ()  [unwired: 2 in, 2 out]
        n181 = property on="Image" class="ImageControl"("16-bit Display Conversion Method"=w409) -> ()  [unwired: 2 in, 2 out]
        n182 = local write "Display Mapping"(w409) -> ()
        n183 = local write "Image"(w398) -> ()
        n184 = local write "Path"(path "" ("Path")) -> ()
        n185 = property on="Image" class="ImageControl"("Zoom to Fit Mode"=TRUE) -> ()  [unwired: 2 in, 2 out]
        n186 = call <vilib>:"Add State(s) to Queue__JKI_lib_State_Machine.vi"("State(s) in Front (\"\")"="UI: Tutorial\n// UI: Progress >> Hide" ("State(s) in Front (\"\")"), "State(s) in (\"\")"=w414) -> ("States Out"=w413:string)  [unwired: 13 in]
      }
      frame "UI: Tutorial" {
        # "Initialize the User Interface, here.\n(this is called automatically, by the Macro: Init)"
        n187 = local read "State"() -> (w429:i32)
        n188 = case shown="8" w429 {
          tunnel: ["Load Calibration Image." "Select a Display Mapping that shows a clear image.\n\nSelect correct PCR size." w448 w466 w473 w480 "Select Well Radius so the center of each well is covered.\n\nGo to previous steps to adjust positions. Press done once satisfied." "Zoom in on Cavity Selection.\n\nEach pixel's temperature is now displayed."] -> w428
          tunnel: [_ _ _ _ _ _ w485 _] -> w427
          tunnel: [_ _ _ _ _ _ w485 _] -> w426
          tunnel: [_ w441 _ _ _ _ _ _] -> w425
          tunnel: [_ w441 _ _ _ _ _ _] -> w424
          tunnel: [w433 w441 w449 w463 w470 w477 _ _] -> w423
          tunnel: [_ w441 w455 w461 w467 w475 w485 w488] -> w422
          tunnel: [TRUE _ _ _ _ _ _ _] -> w421
          tunnel: [_ _ w446 _ _ _ _ w488] -> w420
          tunnel: w419 -> [_ _ w458 w464 w471 w478 _ _]
          tunnel: ["Step: 1/7" "Step: 2/7" "Step: 3/7" "Step: 4/7" "Step: 5/7" "Step: 6/7" "Step: 7/7" "Step: 8/7"] -> w418
          tunnel: [_ _ _ _ _ _ w483 _] -> w417
          tunnel: [_ TRUE w455 w461 w467 w475 TRUE TRUE] -> w416
          tunnel: [_ 0 ("t") w452 3 ("t") 4 ("t") 5 ("t") 6 ("t") 1 ("t")] -> w415
          frame 0, Default {
            n189 = local read "Path"() -> (w435:path)
            n190 = Empty String/Path?(string/path=w435) -> (empty?=w434:bool)
            n191 = Not(x=w434) -> (.not. x?=w433:bool)
          }
          frame 1 {
            w441 = TRUE
          }
          frame 2 {
            w455 = TRUE
            w459 = "Select Fix Point Cavity (Left Click) as shown (zoom with Mouse Wheel).\n\n"  # Select Fix Point Cavity (Left Click) as shown (zoom with Mouse Wheel).
            n192 = Unbundle By Name(w458) -> ("Points.Fixpoint.X"=w457:sgl)
            n193 = local read "Fixpoint Radius"() -> (w451:i32)
            n194 = Not Equal To 0?(x=w457) -> (x != 0?=w446:bool)
            n195 = Not Equal To 0?(x=w451) -> (x != 0?=w450:bool)
            n196 = And(x=w450, y=w446) -> (x .and. y?=w449:bool)
            n197 = Select(t="Set Fixpoint Radius so the cavity is appropriately filled as shown. ", s=w446, f="") -> (s? t:f=w447:string)
            n198 = Select(t=2, s=w446, f=1) -> (s? t:f=w452:i32)
            n199 = Concatenate Strings(w459, w447) -> (w448:string)
          }
          frame 3 {
            w461 = TRUE
            w466 = "Select Top Left corner of PCR plate as shown."  # Select Top Left corner of PCR plate as shown.
            n200 = Unbundle By Name(w464) -> ("Points.Top Left.X"=w465:sgl)
            n201 = Not Equal To 0?(x=w465) -> (x != 0?=w463:bool)
          }
          frame 4 {
            w467 = TRUE
            w473 = "Select Top Right corner of PCR plate as shown."  # Select Top Right corner of PCR plate as shown.
            n202 = Unbundle By Name(w471) -> ("Points.Top Right.X"=w472:sgl)
            n203 = Not Equal To 0?(x=w472) -> (x != 0?=w470:bool)
          }
          frame 5 {
            w475 = TRUE
            w480 = "Select Bottom Left corner of PCR plate as shown."  # Select Bottom Left corner of PCR plate as shown.
            n204 = Unbundle By Name(w478) -> ("Points.Bottom Left.X"=w479:sgl)
            n205 = Not Equal To 0?(x=w479) -> (x != 0?=w477:bool)
          }
          frame 6 {
            w485 = TRUE
            n206 = local read "Well Radius"() -> (w484:u32)
            n207 = Not Equal To 0?(x=w484) -> (x != 0?=w483:bool)
          }
          frame 8 {
            w488 = TRUE
          }
        }
        "Tutorial" <- w428
        "Step" <- w418
        "Pict Ring" <- w415
        n208 = property on="Fixpoint Radius" class="DigNum (strict)"("Visible"=w420) -> ()  [unwired: 2 in, 2 out]
        n209 = property on="Path" class="Path"("Visible"=w421) -> ()  [unwired: 2 in, 2 out]
        n210 = property on="Well Radius" class="DigNum (strict)"("Visible"=w427) -> ()  [unwired: 2 in, 2 out]
        n211 = property on="Show All Points" class="Bool (strict)"("Visible"=w426) -> ()  [unwired: 2 in, 2 out]
        n212 = property on="Display Mapping" class="Ring (strict)"("Visible"=w425) -> ()  [unwired: 2 in, 2 out]
        n213 = property on="PCR Size" class="Ring (strict)"("Visible"=w424) -> ()  [unwired: 2 in, 2 out]
        n214 = property on="Next" class="Bool"("Visible"=w423) -> ()  [unwired: 2 in, 2 out]
        n215 = property on="Previous" class="Bool"("Visible"=w422) -> ()  [unwired: 2 in, 2 out]
        n216 = property on="Save" class="Bool"("Visible"=w417) -> ()  [unwired: 2 in, 2 out]
        n217 = property on="Pict Ring" class="Ring (strict)"("Visible"=w416) -> ()  [unwired: 2 in, 2 out]
        n218 = call <vilib>:"Add State(s) to Queue__JKI_lib_State_Machine.vi"("State(s) in (\"\")"=w432) -> ("States Out"=w431:string)  [unwired: 14 in]
      }
      frame "UI: Cursor Set" {
        # "Argument"
        # "Set and Unset Cursor Busy.\n(Usage: \"UI: Cursor Set >> Busy|Idle\")"
        n219 = case shown="\"Busy\"" w493 {
          tunnel: w495 -> [w500 w502]
          tunnel: [w499 w501] -> w494
          frame "Idle", Default {
            n220 = call <vilib>:"Unset Busy.vi"("error in (no error)"=w500) -> ("error out"=w499:errorcluster)  [unwired: 10 in]
          }
          frame "Busy" {
            n221 = call <vilib>:"Set Busy.vi"("error in (no error)"=w502) -> ("error out"=w501:errorcluster)  [unwired: 9 in, 1 out]
          }
        }
        n222 = call <vilib>:"Add State(s) to Queue__JKI_lib_State_Machine.vi"("State(s) in (\"\")"=w498) -> ("States Out"=w497:string)  [unwired: 14 in]
      }
      frame "UI: Front Panel State" {
        # "Argument"
        # "Set Front Panel Open or Closed\n(Usage: \"UI: Front Panel State >> Open|Close\")"
        n223 = Unbundle By Name(w505) -> ("Core.Current VI Reference"=w504:refnum<vi>)
        n224 = case shown="\"Close\", \"Closed\"" w503 {
          tunnel: w507 -> [w515 w530 w541 w554 w567]
          tunnel: [w517 w531 w543 w556 w569] -> w506
          tunnel: w504 -> [w516 w528 w542 w555 w568]
          frame "Open", "Standard", Default {
            w510 = T5."Standard" ("State")
            n225 = property class="VI"(reference=w516, error in=w515) -> (reference out=w513:refnum<vi>, error out=w514:errorcluster, "FP.State"=w512:T5)
            n226 = Not Equal?(x=w512, y=w510) -> (x != y?=w511:bool)
            n227 = case shown="True" w511 {
              tunnel: [w521 w523] -> w517
              tunnel: w514 -> [w520 w523]
              tunnel: w513 -> [w519 _]
              tunnel: w510 -> [w518 _]
              frame True {
                n228 = invoke class="VI" method="FP.Open"(reference=w519, error in=w520, "Activate"=TRUE, "State"=w518) -> (error out=w521:errorcluster)  [unwired: 1 in, 4 out]
              }
              frame False {
              }
            }
          }
          frame "Close", "Closed" {
            n229 = property class="VI"(reference=w528, error in=w530) -> (reference out=w527:refnum<vi>, error out=w529:errorcluster, "FP.State"=w525:T5)
            n230 = Not Equal?(x=w525, y=T5."Closed" ("Front Panel Window:State")) -> (x != y?=w524:bool)
            n231 = case shown="True" w524 {
              tunnel: [w532 w535] -> w531
              tunnel: w529 -> [w532 w534]
              tunnel: w527 -> [_ w533]
              frame False {
              }
              frame True {
                n232 = invoke class="VI" method="FP.Close"(reference=w533, error in=w534) -> (error out=w535:errorcluster)  [unwired: 1 in, 2 out]
              }
            }
          }
          frame "Hidden", "Hide" {
            w536 = T5."Hidden" ("State")
            n233 = property class="VI"(reference=w542, error in=w541) -> (reference out=w539:refnum<vi>, error out=w540:errorcluster, "FP.State"=w538:T5)
            n234 = Not Equal?(x=w538, y=w536) -> (x != y?=w537:bool)
            n235 = case shown="True" w537 {
              tunnel: [w547 w548] -> w543
              tunnel: w540 -> [w546 w548]
              tunnel: w539 -> [w545 _]
              tunnel: w536 -> [w544 _]
              frame True {
                n236 = invoke class="VI" method="FP.Open"(reference=w545, error in=w546, "State"=w544) -> (error out=w547:errorcluster)  [unwired: 2 in, 4 out]
              }
              frame False {
              }
            }
          }
          frame "Minimize", "Minimized" {
            w549 = T5."Minimized" ("State")
            n237 = property class="VI"(reference=w555, error in=w554) -> (reference out=w552:refnum<vi>, error out=w553:errorcluster, "FP.State"=w551:T5)
            n238 = Not Equal?(x=w551, y=w549) -> (x != y?=w550:bool)
            n239 = case shown="True" w550 {
              tunnel: [w560 w561] -> w556
              tunnel: w553 -> [w559 w561]
              tunnel: w552 -> [w558 _]
              tunnel: w549 -> [w557 _]
              frame True {
                n240 = invoke class="VI" method="FP.Open"(reference=w558, error in=w559, "State"=w557) -> (error out=w560:errorcluster)  [unwired: 2 in, 4 out]
              }
              frame False {
              }
            }
          }
          frame "Maximize", "Maximized" {
            w562 = T5."Maximized" ("State")
            n241 = property class="VI"(reference=w568, error in=w567) -> (reference out=w565:refnum<vi>, error out=w566:errorcluster, "FP.State"=w564:T5)
            n242 = Not Equal?(x=w564, y=w562) -> (x != y?=w563:bool)
            n243 = case shown="True" w563 {
              tunnel: [w573 w574] -> w569
              tunnel: w566 -> [w572 w574]
              tunnel: w565 -> [w571 _]
              tunnel: w562 -> [w570 _]
              frame True {
                n244 = invoke class="VI" method="FP.Open"(reference=w571, error in=w572, "State"=w570) -> (error out=w573:errorcluster)  [unwired: 2 in, 4 out]
              }
              frame False {
              }
            }
          }
        }
        n245 = call <vilib>:"Add State(s) to Queue__JKI_lib_State_Machine.vi"("State(s) in (\"\")"=w509) -> ("States Out"=w508:string)  [unwired: 14 in]
      }
      frame "---------- Macro ----------" {
        # "Do not put any code in this frame.\n(It is a separator no-op. You can make a copy of this frame to create a new Macro frame)"
        n246 = call <vilib>:"Add State(s) to Queue__JKI_lib_State_Machine.vi"("State(s) in (\"\")"=w578) -> ("States Out"=w577:string)  [unwired: 14 in]
      }
      frame "Macro: Initialize" {
        w579 = "// UI: Cursor Set >> Busy\nData: Initialize\nInitialize Core Data\nUI: Initialize\nUI: Front Panel State >> Show\nUI: Tutorial\nData: Load Image\n// Image: Draw\n// UI: Cursor Set >> Idle"  # // UI: Cursor Set >> Busy Data: Initialize Initialize Core Data UI: Initialize UI: Front Panel State >> Show UI: Tutorial Data: Load Image // Image: Draw // UI: Cursor Set >> Idle
        # "Initialization Macro\n(This is called once, when the VI starts)"
        n247 = call <vilib>:"Add State(s) to Queue__JKI_lib_State_Machine.vi"("State(s) in Front (\"\")"=w579, "State(s) in (\"\")"=w583) -> ("States Out"=w582:string)  [unwired: 13 in]
      }
      frame "Macro: Exit" {
        # "Exit Macro\n(This is called once, when the VI exits)"
        n248 = Unbundle By Name(w591) -> ("Core.Close Panel on Exit?"=w590:bool)
        n249 = Select(t="UI: Front Panel State >> Close", s=w590, f="") -> (s? t:f=w587:string)
        n250 = call <vilib>:"Add State(s) to Queue__JKI_lib_State_Machine.vi"("State(s) in Front (\"\")"="Data: Cleanup" ("State(s) in Front (\"\")"), "State(s) in (\"\")"=w587, "State(s) at Back (\"\")"="Exit") -> ("States Out"=w585:string)  [unwired: 12 in]
        n251 = call <vilib>:"Add State(s) to Queue__JKI_lib_State_Machine.vi"("State(s) in Front (\"\")"=w585, "State(s) in (\"\")"=w594) -> ("States Out"=w593:string)  [unwired: 13 in]
      }
      frame "---------- Image ----------" {
        # "Template Separator\n(You can make a copy of, or modify, this frame)"
        n252 = call <vilib>:"Add State(s) to Queue__JKI_lib_State_Machine.vi"("State(s) in (\"\")"=w598) -> ("States Out"=w597:string)  [unwired: 14 in]
      }
      frame "Image: Draw" {
        # "Template Separator\n(You can make a copy of, or modify, this frame)"
        n253 = call <vilib>:"Add State(s) to Queue__JKI_lib_State_Machine.vi"("State(s) in Front (\"\")"="UI: Cursor Set >> Busy\nImage: Clear ROI\nImage: Set ROI\nImage: Draw Fixedpoint\nImage: Calculate BR\nImage: Calculate y space\nImage: Calculate x space\nImage: Calculate Positions\nImage: Drawlines\nImage: Draw Points\nImage: Overlay Cavity Temps\nImage: Overlay Points Temps\nUI: Cursor Set >> Idle" ("State(s) in Front (\"\")"), "State(s) in (\"\")"=w603) -> ("States Out"=w602:string)  [unwired: 13 in]
      }
      frame "Image: Redraw" {
        # "Template Separator\n(You can make a copy of, or modify, this frame)"
        n254 = call <vilib>:"Add State(s) to Queue__JKI_lib_State_Machine.vi"("State(s) in Front (\"\")"="UI: Cursor Set >> Busy\nImage: Clear ROI\nImage: Drawlines\nImage: Draw Points\nImage: Overlay Cavity Temps\nUI: Cursor Set >> Idle" ("State(s) in Front (\"\")"), "State(s) in (\"\")"=w608) -> ("States Out"=w607:string)  [unwired: 13 in]
      }
      frame "Image: Drawlines" {
        # "Template Separator\n(You can make a copy of, or modify, this frame)"
        n255 = Unbundle By Name(w609) -> ("Points.Top Left.X"=w625:sgl, "Points.Top Right.X"=w624:sgl, "Points.Bottom Left.X"=w623:sgl, "Points.Bottom Right.X"=w622:sgl)
        n256 = Equal To 0?(x=w622) -> (x = 0?=w612:bool)
        n257 = Equal To 0?(x=w623) -> (x = 0?=w611:bool)
        n258 = Or(x=w611, y=w612) -> (x .or. y?=w610:bool)
        n259 = Equal To 0?(x=w625) -> (x = 0?=w621:bool)
        n260 = Equal To 0?(x=w624) -> (x = 0?=w620:bool)
        n261 = Select(t="", s=w611, f="Image: Draw Line >> TL_BL\n") -> (s? t:f=w617:string)
        n262 = Select(t="", s=w610, f="Image: Draw Line >> TR_BR\nImage: Draw Line >> BL_BR\nImage: Draw Line >> Vertical\nImage: Draw Line >> Horizontal") -> (s? t:f=w614:string)
        n263 = case shown="False" w621 {
          tunnel: w620 -> [w632 _]
          tunnel: w617 -> [w631 _]
          tunnel: w614 -> [w630 _]
          tunnel: [w629 _] -> w613
          frame False {
            n264 = case shown="False" w632 {
              tunnel: w631 -> [w635 _]
              tunnel: w630 -> [w634 _]
              tunnel: [w633 _] -> w629
              frame False {
                n265 = Concatenate Strings("Image: Draw Line >> TL_TR\n", w635, w634) -> (w633:string)
              }
              frame True {
              }
            }
          }
          frame True {
          }
        }
        n266 = call <vilib>:"Add State(s) to Queue__JKI_lib_State_Machine.vi"("State(s) in Front (\"\")"=w613, "State(s) in (\"\")"=w628) -> ("States Out"=w627:string)  [unwired: 13 in]
      }
      frame "Image: Draw Fixedpoint" {
        # "Template Separator\n(You can make a copy of, or modify, this frame)"
        n267 = Unbundle By Name(w643) -> ("Image Out"=w640:T2, "Points.Fixpoint"=w642:T3)
        n268 = Build Array(w642) -> (w641:T3[])
        n269 = call "TCam_CenterArray.vi"("Image in"=w640, "Point Array"=w641, "Size"="Fixpoint Radius") -> ("Image"=w639:T2)  [unwired: 3 in, 2 out]
        n270 = local write "Image"(w639) -> ()
        n271 = call <vilib>:"Add State(s) to Queue__JKI_lib_State_Machine.vi"("State(s) in (\"\")"=w645) -> ("States Out"=w644:string)  [unwired: 14 in]
      }
      frame "Image: Overlay Cavity Temps" {
        # "Template Separator\n(You can make a copy of, or modify, this frame)"
        n272 = local read "OverlayTemp"() -> (w646:bool)
        n273 = case shown="True" w646 {
          tunnel: w648 -> [_ w658]
          frame False {
          }
          frame True {
            n274 = local read "Fixpoint Radius"() -> (w654:i32)
            n275 = Unbundle By Name(w658) -> ("Image Out"=w655:T2, "Points.Fixpoint"=w657:T3)
            n276 = Build Array(w657) -> (w656:T3[])
            n277 = call "TCam_CenterArray.vi"("Image in"=w655, "Point Array"=w656, "Size"=w654) -> ("Image"=w651:T2, "Array"=w653:cluster{"X":i32, "Y":i32}[][])  [unwired: 3 in, 1 out]
            n278 = call "OverlayTemps.vi"("Points"=w653, "Image"=w651) -> ("Image Out"=w652:T2)  [unwired: 9 in]
            n279 = local write "Image"(w652) -> ()
          }
        }
        n280 = call <vilib>:"Add State(s) to Queue__JKI_lib_State_Machine.vi"("State(s) in (\"\")"=w650) -> ("States Out"=w649:string)  [unwired: 14 in]
      }
      frame "Image: Clear ROI" {
        # "Your code here.\n(You can make a copy of, or modify, this frame)"
        n281 = Unbundle By Name(w662) -> ("Image Out"=w661:T2)
        n282 = call "IMAQ Clear Overlay"("error in (no error)"=w660, "Image"=w661) -> ("error out"=w659:errorcluster)  [unwired: 8 in, 1 out]
        n283 = call <vilib>:"Add State(s) to Queue__JKI_lib_State_Machine.vi"("State(s) in (\"\")"=w664) -> ("States Out"=w663:string)  [unwired: 14 in]
      }
      frame "Image: Calculate x space" {
        # "Your code here.\n(You can make a copy of, or modify, this frame)"
        n284 = Unbundle By Name(w673) -> ("Points.Top Left"=w679:T3, "Points.Top Right"=w678:T3)
        n285 = case shown="1" "PCR Size" {
          tunnel: [24 12] -> w665
          frame 0, Default {
          }
          frame 1 {
          }
        }
        n286 = Unbundle(w678) -> ("X"=w677:sgl, "Y"=w675:sgl)
        n287 = Unbundle(w679) -> ("X"=w676:sgl, "Y"=w674:sgl)
        n288 = Subtract(x=w677, y=w676) -> (x-y=w670:sgl)
        n289 = Decrement(x=w665) -> (x-1=w669:i32)
        n290 = Subtract(x=w675, y=w674) -> (x-y=w668:sgl)
        n291 = Divide(x=w670, y=w669) -> (x/y=w671:sgl)
        n292 = Divide(x=w668, y=w669) -> (x/y=w667:sgl)
        n293 = Bundle By Name(cluster=w673, "Points.x_space"=w671, "Points.y_space"=w667) -> (w672:T1)
        n294 = call <vilib>:"Add State(s) to Queue__JKI_lib_State_Machine.vi"("State(s) in (\"\")"=w682) -> ("States Out"=w681:string)  [unwired: 14 in]
      }
      frame "Image: Calculate BR" {
        # "Your code here.\n(You can make a copy of, or modify, this frame)"
        n295 = Unbundle By Name(w693) -> ("Points.Top Left"=w699:T3, "Points.Top Right"=w698:T3, "Points.Bottom Left"=w691:T3)
        n296 = Unbundle(w699) -> ("X"=w696:sgl, "Y"=w694:sgl)
        n297 = Unbundle(w698) -> ("X"=w697:sgl, "Y"=w695:sgl)
        n298 = Unbundle(w691) -> ("X"=w690:sgl, "Y"=w688:sgl)
        n299 = Subtract(x=w697, y=w696) -> (x-y=w689:sgl)
        n300 = Subtract(x=w695, y=w694) -> (x-y=w687:sgl)
        n301 = Add(x=w690, y=w689) -> (x+y=w685:sgl)
        n302 = Add(x=w687, y=w688) -> (x+y=w686:sgl)
        n303 = Bundle By Name(cluster=w693, "Points.Bottom Right.X"=w685, "Points.Bottom Right.Y"=w686) -> (w692:T1)
        n304 = call <vilib>:"Add State(s) to Queue__JKI_lib_State_Machine.vi"("State(s) in (\"\")"=w702) -> ("States Out"=w701:string)  [unwired: 14 in]
      }
      frame "Image: Calculate y space" {
        # "Your code here.\n(You can make a copy of, or modify, this frame)"
        n305 = local read "PCR Size"() -> (w704:u16)
        n306 = Unbundle By Name(w711) -> ("Points.Top Left"=w717:T3, "Points.Bottom Left"=w716:T3)
        n307 = case shown="1" w704 {
          tunnel: [16 8] -> w703
          frame 0, Default {
          }
          frame 1 {
          }
        }
        n308 = Unbundle(w716) -> ("X"=w715:sgl, "Y"=w713:sgl)
        n309 = Unbundle(w717) -> ("X"=w714:sgl, "Y"=w712:sgl)
        n310 = Subtract(x=w715, y=w714) -> (x-y=w708:sgl)
        n311 = Decrement(x=w703) -> (x-1=w707:i32)
        n312 = Subtract(x=w713, y=w712) -> (x-y=w706:sgl)
        n313 = Divide(x=w708, y=w707) -> (x/y=w709:sgl)
        n314 = Divide(x=w706, y=w707) -> (x/y=w705:sgl)
        n315 = Bundle By Name(cluster=w711, "Points.x space 2"=w709, "Points.y space 2"=w705) -> (w710:T1)
        n316 = call <vilib>:"Add State(s) to Queue__JKI_lib_State_Machine.vi"("State(s) in (\"\")"=w720) -> ("States Out"=w719:string)  [unwired: 14 in]
      }
      frame "Image: Set ROI" {
        # "Your code here.\n(You can make a copy of, or modify, this frame)"
        n317 = Unbundle By Name(w729) -> ("State"=w727:i32)
        n318 = case shown="2..5" w727 {
          tunnel: w727 -> [_ w741]
          tunnel: w729 -> [_ w739]
          tunnel: w728 -> [w734 w738]
          tunnel: [w734 w737] -> w726
          tunnel: [T12 {"Global Rectangle"=[], "Contours"=[]} ("ROI Descriptor") w736] -> w725
          tunnel: [w732 w735] -> w723
          frame 0, Default {
            w732 = u32 0 items=["Zoom Tool"=8, "Selection Tool"=0, "Pan Tool"=9, "Point Tool"=1, "Line Tool"=2, "Rectangle Tool"=3, "Rotated Rectangle Tool"=12, "Polyline Tool"=10, "Polygon Tool"=5, "Freehand Tool"=11, "Closed Freehand Tool"=6, "Ellipse Tool"=4, "Annulus Tool"=7] ("Current ROI Tool")
          }
          frame 2..5 {
            w735 = u32 1 items=["Zoom Tool"=8, "Selection Tool"=0, "Pan Tool"=9, "Point Tool"=1, "Line Tool"=2, "Rectangle Tool"=3, "Rotated Rectangle Tool"=12, "Polyline Tool"=10, "Polygon Tool"=5, "Freehand Tool"=11, "Closed Freehand Tool"=6, "Ellipse Tool"=4, "Annulus Tool"=7] ("Current ROI Tool")
            n319 = case shown="5" w741 {
              tunnel: [w743 w745 w747 w749] -> w740
              tunnel: w739 -> [w742 w744 w746 w748]
              frame 2, Default {
                n320 = Unbundle By Name(w742) -> ("Points.Fixpoint"=w743:T3)
              }
              frame 3 {
                n321 = Unbundle By Name(w744) -> ("Points.Top Left"=w745:T3)
              }
              frame 4 {
                n322 = Unbundle By Name(w746) -> ("Points.Top Right"=w747:T3)
              }
              frame 5 {
                n323 = Unbundle By Name(w748) -> ("Points.Bottom Left"=w749:T3)
              }
            }
            n324 = call "IMAQ Convert Point to ROI"("error in (no error)"=w738, "Point"=w740) -> ("error out"=w737:errorcluster, "ROI Descriptor"=w736:T12)  [unwired: 7 in]
          }
        }
        n325 = property on="Image" class="ImageControl"("Current ROI Tool"=w723) -> ()  [unwired: 2 in, 2 out]
        n326 = property on="Image" class="ImageControl"(error in=w726, "ROI"=w725) -> (error out=w724:errorcluster)  [unwired: 1 in, 1 out]
        n327 = call <vilib>:"Add State(s) to Queue__JKI_lib_State_Machine.vi"("State(s) in (\"\")"=w731) -> ("States Out"=w730:string)  [unwired: 14 in]
      }
      frame "Image: Draw Line" {
        w750 = u32 1  # Width_Minor
        w751 = u32 2  # Width
        # "Your code here.\n(You can make a copy of, or modify, this frame)"
        n328 = Unbundle By Name(w755) -> ("Image Out"=w756:T2)
        n329 = case shown="\"False\", Default" w757 {
          tunnel: w756 -> [w761 w769 w778 w785 w791 w796 w805]
          tunnel: w755 -> [_ w770 w779 w781 w787 w800 w809]
          tunnel: [w761 w764 w777 w784 w790 w792 w801] -> w754
          tunnel: w753 -> [w760 w768 w776 w783 w789 w794 w804]
          tunnel: [w760 w763 w775 w782 w788 w793 w803] -> w752
          tunnel: w751 -> [_ w762 w771 _ _ w795 w802]
          tunnel: w750 -> [_ _ _ w780 w786 _ _]
          frame "False", Default {
          }
          frame "TL_TR" {
            n330 = Unbundle By Name(w770) -> ("Points.Top Left"=w767:T3, "Points.Top Right"=w766:T3)
            n331 = Build Array(w767, w766) -> (w765:T3[])
            n332 = call "IMAQ Overlay Multiple Lines 2"("Image"=w769, "Line End Points"=w765, "error in (no error)"=w768, "Width"=w762) -> ("Image Out"=w764:T2, "error out"=w763:errorcluster)  [unwired: 10 in]
          }
          frame "TL_BL" {
            n333 = Unbundle By Name(w779) -> ("Points.Top Left"=w774:T3, "Points.Bottom Left"=w773:T3)
            n334 = Build Array(w774, w773) -> (w772:T3[])
            n335 = call "IMAQ Overlay Multiple Lines 2"("Image"=w778, "Line End Points"=w772, "error in (no error)"=w776, "Width"=w771) -> ("Image Out"=w777:T2, "error out"=w775:errorcluster)  [unwired: 10 in]
          }
          frame "Vertical" {
            n336 = call "TCam_VerticalLines.vi"("Width"=w780, "error in (no error)"=w783, "Cluster"=w781, "Refnum in"=w785) -> ("error out"=w782:errorcluster, "Refnum out"=w784:T2)  [unwired: 6 in]
          }
          frame "Horizontal" {
            n337 = call "TCam_HorizontalLines.vi"("Width"=w786, "error in (no error)"=w789, "Cluster"=w787, "Refnum in"=w791) -> ("error out"=w788:errorcluster, "Refnum out"=w790:T2)  [unwired: 6 in]
          }
          frame "TR_BR" {
            n338 = Unbundle By Name(w800) -> ("Points.Top Right"=w799:T3, "Points.Bottom Right"=w798:T3)
            n339 = Build Array(w799, w798) -> (w797:T3[])
            n340 = call "IMAQ Overlay Multiple Lines 2"("Image"=w796, "Line End Points"=w797, "error in (no error)"=w794, "Width"=w795) -> ("Image Out"=w792:T2, "error out"=w793:errorcluster)  [unwired: 10 in]
          }
          frame "BL_BR" {
            n341 = Unbundle By Name(w809) -> ("Points.Bottom Left"=w808:T3, "Points.Bottom Right"=w807:T3)
            n342 = Build Array(w808, w807) -> (w806:T3[])
            n343 = call "IMAQ Overlay Multiple Lines 2"("Image"=w805, "Line End Points"=w806, "error in (no error)"=w804, "Width"=w802) -> ("Image Out"=w801:T2, "error out"=w803:errorcluster)  [unwired: 10 in]
          }
        }
        n344 = local write "Image"(w754) -> ()
        n345 = call <vilib>:"Add State(s) to Queue__JKI_lib_State_Machine.vi"("State(s) in (\"\")"=w759) -> ("States Out"=w758:string)  [unwired: 14 in]
      }
      frame "Image: Draw Points" {
        # "Your code here.\n(You can make a copy of, or modify, this frame)"
        n346 = Unbundle By Name(w811) -> ("Points.Top Left.X"=w820:sgl, "Points.Top Right.X"=w819:sgl, "Points.Bottom Left.X"=w818:sgl, "Points.Bottom Right.X"=w817:sgl)
        n347 = Equal To 0?(x=w820) -> (x = 0?=w816:bool)
        n348 = Equal To 0?(x=w819) -> (x = 0?=w815:bool)
        n349 = Equal To 0?(x=w818) -> (x = 0?=w814:bool)
        n350 = Equal To 0?(x=w817) -> (x = 0?=w813:bool)
        n351 = Unbundle By Name(w811) -> ("Image Out"=w822:T2)
        n352 = Compound Arithmetic op=OR(w816, w815, w814, w813) -> (w812:bool)
        n353 = case shown="False" w812 {
          tunnel: w822 -> [w832 _]
          tunnel: w811 -> [w827 w833]
          tunnel: [w825 w833] -> w810
          frame False {
            n354 = local read "Points"() -> (w831:T3[])
            n355 = call "TCam_CenterArray.vi"("Image in"=w832, "Point Array"=w831, "Size"="Well Radius", "draw all?"="Show All Points") -> ("Image"=w829:T2, "Array"=w826:cluster{"X":i32, "Y":i32}[][])  [unwired: 2 in, 1 out]
            n356 = local write "Image"(w829) -> ()
            n357 = Bundle By Name(cluster=w827, "Points.Pixels"=w826) -> (w825:T1)
          }
          frame True {
          }
        }
        n358 = call <vilib>:"Add State(s) to Queue__JKI_lib_State_Machine.vi"("State(s) in (\"\")"=w824) -> ("States Out"=w823:string)  [unwired: 14 in]
      }
      frame "Image: Overlay Points Temps" {
        # "Your code here.\n(You can make a copy of, or modify, this frame)"
        n359 = local read "OverlayTemp"() -> (w835:bool)
        n360 = case shown="True" w835 {
          tunnel: w834 -> [_ w839]
          frame False {
          }
          frame True {
            n361 = Unbundle By Name(w839) -> ("Points.Top Left.X"=w848:sgl, "Points.Top Right.X"=w847:sgl, "Points.Bottom Left.X"=w846:sgl, "Points.Bottom Right.X"=w845:sgl)
            n362 = Unbundle By Name(w839) -> ("Image Out"=w849:T2)
            n363 = Equal To 0?(x=w848) -> (x = 0?=w844:bool)
            n364 = Equal To 0?(x=w847) -> (x = 0?=w843:bool)
            n365 = Equal To 0?(x=w846) -> (x = 0?=w842:bool)
            n366 = Equal To 0?(x=w845) -> (x = 0?=w841:bool)
            n367 = Compound Arithmetic op=OR(w844, w843, w842, w841) -> (w840:bool)
            n368 = case shown="False" w840 {
              tunnel: w849 -> [w856 _]
              frame False {
                n369 = local read "Well Radius"() -> (w854:u32)
                n370 = local read "Points"() -> (w855:T3[])
                n371 = local read "Show All Points"() -> (w853:bool)
                n372 = call "TCam_CenterArray.vi"("Image in"=w856, "Point Array"=w855, "Size"=w854, "draw all?"=w853) -> ("Image"=w852:T2, "Points"=w851:cluster{"X":i32, "Y":i32}[][])  [unwired: 2 in, 1 out]
                n373 = call "OverlayTemps.vi"("Points"=w851, "Image"=w852) -> ("Image Out"=w850:T2)  [unwired: 9 in]
                n374 = local write "Image"(w850) -> ()
              }
              frame True {
              }
            }
          }
        }
        n375 = call <vilib>:"Add State(s) to Queue__JKI_lib_State_Machine.vi"("State(s) in (\"\")"=w838) -> ("States Out"=w837:string)  [unwired: 14 in]
      }
      frame "Image: Calculate Positions" {
        # "Your code here.\n(You can make a copy of, or modify, this frame)"
        n376 = Unbundle By Name(w858) -> ("Points.Top Left.X"=w866:sgl, "Points.Top Right.X"=w865:sgl, "Points.Bottom Left.X"=w864:sgl, "Points.Bottom Right.X"=w863:sgl)
        n377 = Equal To 0?(x=w866) -> (x = 0?=w862:bool)
        n378 = Equal To 0?(x=w865) -> (x = 0?=w861:bool)
        n379 = Equal To 0?(x=w864) -> (x = 0?=w860:bool)
        n380 = Equal To 0?(x=w863) -> (x = 0?=w859:bool)
        n381 = Compound Arithmetic op=OR(w862, w861, w860, w859) -> (w857:bool)
        n382 = case shown="False" w857 {
          tunnel: w858 -> [w870 _]
          frame False {
            n383 = local read "PCR Size"() -> (w871:u16)
            n384 = call "TCam_PointCalculator.vi"("Cluster"=w870, "Size"=w871) -> ("Points"=→"Points":T3[])  [unwired: 9 in]
          }
          frame True {
          }
        }
        n385 = call <vilib>:"Add State(s) to Queue__JKI_lib_State_Machine.vi"("State(s) in (\"\")"=w869) -> ("States Out"=w868:string)  [unwired: 14 in]
      }
    }
  }
  "State out" <- "Data: Load Thermal Calibration"
